vi "探头数据读取.vi"(11 "编号":string) -> ()   [LabVIEW 2022 SP3, in "斯坦道多参数.lvlib"]
panel:
  out "日期/时间字符串 2":string
  out "日期/时间字符串":string
  out "运行状态":u16(ring) items=["空闲", "水样测试", "标样核查"]
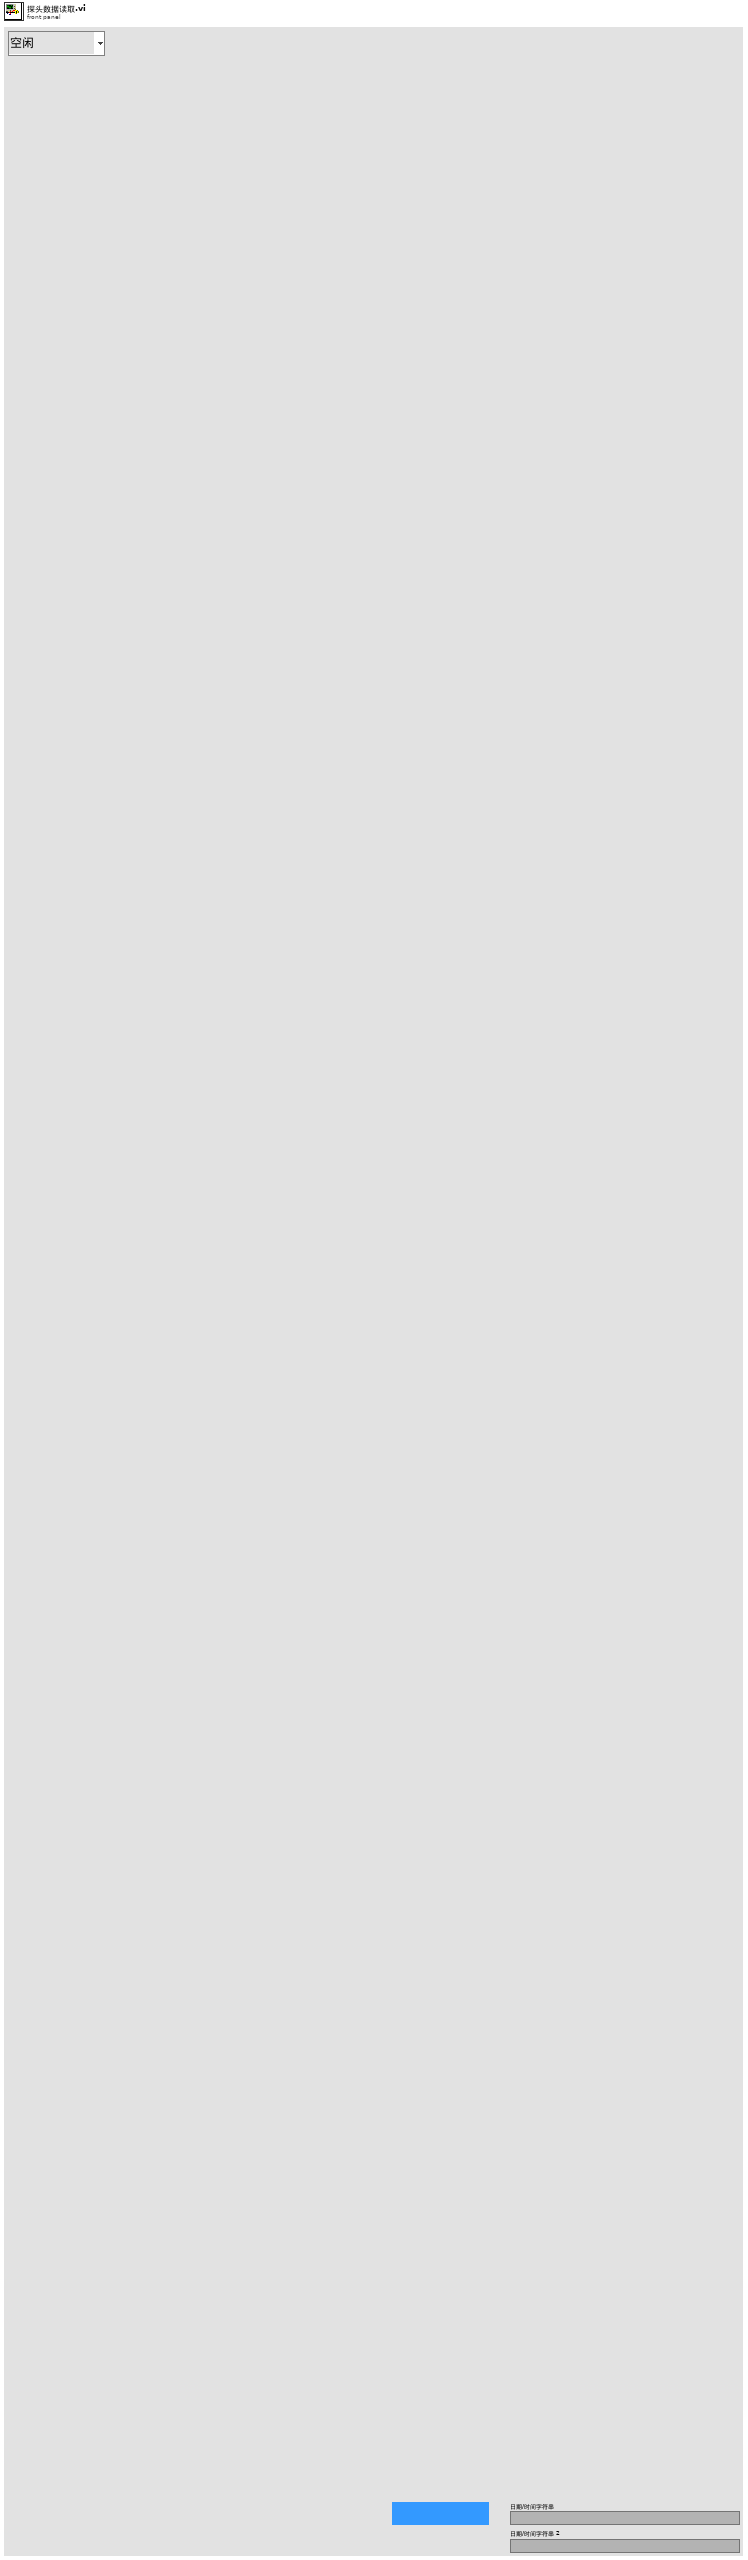
[diagram p1: front panel]
types:
  T1 = typedef "斯坦道多参数.lvlib/通知队列类型.ctl" = enum16{"pH", "DO", "DO2", "Cond", "Turb", "ORP", "叶绿素a", "藻密度", "COD", "氯化物", "氨氮", "水中油", "悬浮物", "余氯"}
  T2 = cluster{"温度测量值":sgl, "测量值":sgl, "温度偏移修正值":sgl, "信号值":sgl, "数据标识":string}
  T3 = cluster{"温度测量值":sgl, "DO%":sgl, "DOmg/L":sgl, "温度偏移修正值":sgl, "数据标识mg/L":string, "数据标识%":string}
  T4 = cluster{"水温 (℃)":cluster{"量程下限":dbl, "量程上限":dbl}, "DO (mg/L)":cluster{"量程下限":dbl, "量程上限":dbl}, "DO (%)":cluster{"量程下限":dbl, "量程上限":dbl}, "pH":cluster{"量程下限":dbl, "量程上限":dbl}, "电导率 (μS/cm)":cluster{"量程下限":dbl, "量程上限":dbl}, "盐度":cluster{"量程下限":dbl, "量程上限":dbl}, "浊度 (NTU)":cluster{"量程下限":dbl, "量程上限":dbl}, "叶绿素a (μg/L)":cluster{"量程下限":dbl, "量程上限":dbl}, "藻密度 (cells/mL)":cluster{"量程下限":dbl, "量程上限":dbl}, "ORP (mV)":cluster{"量程下限":dbl, "量程上限":dbl}, "氯化物（mg/L）":cluster{"量程下限":dbl, "量程上限":dbl}, "COD":cluster{"量程下限":dbl, "量程上限":dbl}, "氨氮":cluster{"量程下限":dbl, "量程上限":dbl}, "水中油":cluster{"量程下限":dbl, "量程上限":dbl}, "悬浮物":cluster{"量程下限":dbl, "量程上限":dbl}, "余氯":cluster{"量程下限":dbl, "量程上限":dbl}}
  T5 = cluster{"CH":u16, "监测值":dbl, "信号值":sgl, "数据标识":string}
  T6 = typedef "斯坦道多参数.lvlib/探头类型.ctl" = enum16{"禹山", "国弘", "纳清", "STD"}
  T7 = cluster{"pH探头选择":T6, "DO探头选择":T6, "电导率探头选择":T6, "浊度探头选择":T6, "悬浮物探头选择":T6, "叶绿素a探头选择":T6, "蓝绿藻探头选择":T6, "orp探头选择":T6, "COD探头选择":T6, "DO2探头选择":T6, "氨氮探头选择":T6, "水中油探头选择":T6, "余氯探头选择":T6}
  T8 = cluster{"电极状态标志":u16, "电极型号标志":u16, "酸碱度测量值":sgl, "温度测量值":sgl, "酸碱度信号值":sgl, "温度信号值":sgl, "酸碱度偏移修正值":sgl, "温度偏移修正值":sgl, "手动温度补偿值":sgl, "酸碱度电极零点":sgl, "酸碱度电极斜率":sgl, "第1点标准值记录":sgl, "第1点信号值记录":sgl, "第1点温度值记录":sgl, "第2点标准值记录":sgl, "第2点信号值记录":sgl, "第2点温度值记录":sgl, "命令滤波设定":u16, "温度模式":enum16{"ATC", "MTC"}, "生产批次":u16, "电极序号":u16, "串口地址":u16, "串口波特率":enum16{"9600", "19200", "115200"}, "串口校验位":enum16{"NONE", "ODD", "EVEN"}, "串口停止位":enum16{"1bit", "2bit"}, "第一点标准值":sgl, "第二点标准值":sgl}
  T9 = cluster{"报警码":u16, "pH数值":sgl, "0X0003_NC":sgl, "温度数据":sgl, "pH原始信号 mv":sgl, "0X0009_NC":string, "产品名称":string, "序列号":string, "硬件版本":string, "软件版本":string, "通讯地址":u16, "波特率":u16, "设备类型":u16, "0X0026_NC":string, "第一点原始数据":sgl, "第一点校准数据":sgl, "第二点原始数据":sgl, "第二点校准数据":sgl, "探头校准命令":u16, "温度校准参数":sgl, "温度校准命令":u16}
  T10 = cluster{"电极状态标志":u16, "电极型号标志":u16, "电导率测量值":sgl, "温度测量值":sgl, "电导率信号值":sgl, "温度信号值":sgl, "温度补偿系数":sgl, "电导率偏移修正值":sgl, "温度偏移修正值":sgl, "手动温度补偿值":sgl, "电导率电极零点":sgl, "电导率电极斜率":sgl, "命令滤波设定":u16, "温度模式":enum16{"ATC", "MTC"}, "生产批次":u16, "电极序号":u16, "串口地址":u16, "串口波特率":enum16{"9600", "19200", "115200"}, "串口校验位":enum16{"NONE", "ODD", "EVEN"}, "串口停止位":enum16{"1bit", "2bit"}, "第一点标准值":sgl, "第二点标准值":sgl}
  T11 = cluster{"报警码":u16, "电导率数据（uS/cm）":sgl, "0x0003 NC":sgl, "温度数据":sgl, "电导率原始信号电阻":sgl, "当前量程":u16, "温度补偿系数":sgl, "0X0009_NC":string, "产品名称":string, "序列号":string, "硬件版本":string, "软件版本":string, "通讯地址":u16, "波特率":u16, "设备类型":u16, "0X0026_NC":string, "第一点原始数据":sgl, "第一点校准数据":sgl, "0X0035_NC":sgl, "0X0037_NC":sgl, "探头校准命令":u16, "温度校准参数":sgl, "温度校准命令":u16}
  T12 = cluster{"电极状态标志":u16, "电极型号标志":u16, "溶解氧测量值":sgl, "温度测量值":sgl, "溶解氧饱和度值":sgl, "盐度补偿值":sgl, "大气压补偿值":sgl, "溶解氧偏移修正值":sgl, "温度偏移修正值":sgl, "手动温度补偿值":sgl, "溶解氧电极零点":sgl, "溶解氧电极斜率":sgl, "第1点标准值记录":sgl, "第1点信号值记录":sgl, "第1点温度值记录":sgl, "第2点标准值记录":sgl, "第2点信号值记录":sgl, "第2点温度值记录":sgl, "命令滤波设定":u16, "温度模式":enum16{"ATC", "MTC"}, "生产批次":u16, "电极序号":u16, "串口地址":u16, "串口波特率":enum16{"9600", "19200", "115200"}, "串口校验位":enum16{"NONE", "ODD", "EVEN"}, "串口停止位":enum16{"1bit", "2bit"}, "第一点标准值":sgl, "第二点标准值":sgl}
  T13 = cluster{"报警码":u16, "溶解氧数值（mg/L）":sgl, "溶解氧数据（%）":sgl, "温度数据":sgl, "溶解氧原始信号 nA":sgl, "大气压力":sgl, "盐度":sgl, "0X0009_NC":string, "产品名称":string, "序列号":string, "硬件版本":string, "软件版本":string, "通讯地址":u16, "波特率":u16, "设备类型":u16, "0X0026_NC":string, "第一点原始数据":sgl, "0X0033 NC":sgl, "第二点原始数据":sgl, "0X0037 NC":sgl, "探头校准命令":u16, "温度校准参数":sgl, "温度校准命令":u16}
  T14 = cluster{"电极状态标志":u16, "电极型号标志":u16, "浊度测量值":sgl, "温度测量值":sgl, "浊度信号值":sgl, "浊度偏移修正值":sgl, "温度偏移修正值":sgl, "手动温度补偿值":sgl, "浊度电极零点":sgl, "浊度电极斜率":sgl, "清洁周期":u16, "命令滤波设定":u16, "温度模式":enum16{"ATC", "MTC"}, "生产批次":u16, "电极序号":u16, "串口地址":u16, "串口波特率":enum16{"9600", "19200", "115200"}, "串口校验位":enum16{"NONE", "ODD", "EVEN"}, "串口停止位":enum16{"1bit", "2bit"}, "第一点标准值":sgl, "第二点标准值":sgl, "第三点标准值":sgl}
  T15 = cluster{"报警码":u16, "浊度数值 NTU":sgl, "温度数据":sgl, "原始光强数值":u16, "量程":u16, "平均次数":u16, "清扫模式":u16, "清扫次数":u16, "清扫间隔分钟":u16, "0X000B_NC":string, "产品名称":string, "序列号":string, "硬件版本":string, "软件版本":string, "通讯地址":u16, "波特率":u16, "设备类型":u16, "0X0026_NC":string, "校准量程":u16, "第一点原始光强":u16, "第一点校准数据":sgl, "第二点原始光强":u16, "第二点校准数据":sgl, "第三点原始光强":u16, "第三点校准数据":sgl, "探头校准命令":u16, "温度校准参数":sgl, "温度校准命令":u16}
  T16 = cluster{"电极状态标志":u16, "电极型号标志":u16, "测量值":sgl, "温度测量值":sgl, "信号值":sgl, "温度信号值":sgl, "000AH_NC":sgl, "偏移修正值":sgl, "温度偏移修正值":sgl, "手动温度补偿值":sgl, "命令滤波设定":u16, "温度模式":enum16{"ATC", "MTC"}, "生产批次":u16, "传感器序号":u16, "串口地址":u16, "串口波特率":enum16{"9600", "19200", "115200"}, "串口校验位":enum16{"NONE", "ODD", "EVEN"}, "串口停止位":enum16{"1bit", "2bit"}}
  T17 = cluster{"报警码":u16, "叶绿素a":sgl, "温度数据":sgl, "原始光强数值":u16, "量程":u16, "平均次数":u16, "清扫模式":u16, "清扫次数":u16, "清扫间隔分钟":u16, "0X000B_NC":string, "产品名称":string, "序列号":string, "硬件版本":string, "软件版本":string, "通讯地址":u16, "波特率":u16, "设备类型":u16, "0X0026_NC":string, "校准量程":u16, "第一点原始光强":u16, "第一点校准数据":sgl, "第二点原始光强":u16, "第二点校准数据":sgl, "第三点原始光强":u16, "第三点校准数据":sgl, "探头校准命令":u16, "温度校准参数":sgl, "温度校准命令":u16}
  T18 = cluster{"报警码":u16, "蓝绿藻":sgl, "温度数据":sgl, "原始光强数值":u16, "0X0006_NC":u16, "平均次数":u16, "清扫模式":u16, "清扫次数":u16, "清扫间隔分钟":u16, "0X000B_NC":string, "产品名称":string, "序列号":string, "硬件版本":string, "软件版本":string, "通讯地址":u16, "波特率":u16, "设备类型":u16, "0X0026_NC":string, "0X0030_NC":u16, "第一点原始光强":u16, "第一点校准数据":sgl, "第二点原始光强":u16, "第二点校准数据":sgl, "第三点原始光强":u16, "第三点校准数据":sgl, "探头校准命令":u16, "温度校准参数":sgl, "温度校准命令":u16}
  T19 = cluster{"电极状态标志":u16, "电极型号标志":u16, "COD测量值":sgl, "浊度测量值":sgl, "COD信号值":sgl, "浊度信号值":sgl, "温度测量值":sgl, "COD偏移修正值":sgl, "浊度偏移修正值":sgl, "COD水样校正值":sgl, "温度偏移修正值":sgl, "COD零点系数":sgl, "COD斜率系数":sgl, "浊度零点系数":sgl, "浊度斜率系数":sgl, "COD测值K值":sgl, "浊度测值K值":sgl, "浊度补偿COD系数值":sgl, "COD温度补偿系数值 ":sgl, "测量周期":u16, "清洗周期":u16, "命令寄存器":u16, "数字滤波设定":u16, "温度模式":enum16{"AUTO", "OFF"}, "生产批次":u16, "电极序号":u16, "串口地址":u16, "串口波特率":enum16{"9600", "19200", "115200"}, "串口校验位":enum16{"NONE", "ODD", "EVEN"}, "串口停止位":enum16{"1bit", "2bit"}, "第一点校正指令":u16, "第一点标准值":sgl, "第二点校正指令":u16, "第二点标准值":sgl, "第三点校正指令":u16, "第三点标准值":sgl, "COD吸光度":sgl, "浊度吸光度":sgl, "温度信号值":sgl}
  T20 = cluster{"电极状态标志":u16, "电极型号标志":u16, "测量值":sgl, "温度测量值":sgl, "信号值":sgl, "温度信号值":sgl, "偏移修正值":sgl, "温度偏移修正值":sgl, "手动温度补偿值":sgl, "电极零点":sgl, "电极斜率":sgl, "第1点标准值记录":sgl, "第1点信号值记录":sgl, "第1点温度值记录":sgl, "第2点标准值记录":sgl, "第2点信号值记录":sgl, "第2点温度值记录":sgl, "命令滤波设定":u16, "温度模式":enum16{"ATC", "MTC"}, "生产批次":u16, "电极序号":u16, "串口地址":u16, "串口波特率":enum16{"9600", "19200", "115200"}, "串口校验位":enum16{"NONE", "ODD", "EVEN"}, "串口停止位":enum16{"1bit", "2bit"}, "第一点标准值":sgl, "第二点标准值":sgl}
  T21 = cluster{"电极状态标志":u16, "电极型号标志":u16, "测量值":sgl, "温度测量值":sgl, "信号值":sgl, "水中油B值":sgl, "温度B值":sgl, "水中油零点系数":sgl, "水中油斜率系数":sgl, "水中油K值":sgl, "空白电位值":sgl, "温度信号值":sgl, "温度补偿系数":sgl, "测量档位":u16, "清洁周期":u16, "命令寄存器":u16, "数位滤波设定":u16, "温度模式":enum16{"ATC", "MTC"}, "生产批次":u16, "电极序号":u16, "串口地址":u16, "串口波特率":enum16{"9600", "19200", "115200"}, "串口校验位":enum16{"NONE", "ODD", "EVEN"}, "串口停止位":enum16{"1bit", "2bit"}, "第一点校正指令":u16, "第一点标准值":sgl, "第二点校正指令":u16, "第二点标准值":sgl, "第三点校正指令":u16, "第三点标准值":sgl}
  T22 = cluster{"余氯值":sgl, "温度值":sgl, "温度电压_mv":sgl, "氯电压_mv":dbl, "pH补偿值":dbl, "氯偏置":dbl, "温度偏置":dbl, "序列号":string}
  T23 = cluster{"报警码":u16, "参数1数据":sgl, "参数2数据":sgl, "参数3数据":sgl, "参数4数据":sgl, "温度数据":sgl, "参数1原始信号":sgl, "参数2原始信号":sgl, "参数3原始信号":sgl, "参数4原始信号":sgl, "序列号":string, "硬件版本":string, "软件版本":string, "通讯地址":u16, "波特率":u16, "设备类型":u16, "0X0026_NC":string, "校准参数类型":u16, "第一点原始数据":sgl, "第一点校准数据":sgl, "第二点原始数据":sgl, "第二点校准数据":sgl, "探头校准命令":u16, "温度校准参数":sgl, "温度校准命令":u16}
  T24 = cluster{"ph":bool, "DO":bool, "Cond":bool, "Turb":bool, "叶绿素a":bool, "藻密度":bool, "ORP":bool, "cod":bool, "DO2":bool, "氯化物":bool, "氨氮":bool, "水中油":bool, "悬浮物":bool, "余氯":bool}
  T25 = cluster{"ph":bool, "DO":bool, "Cond":bool, "Turb":bool, "叶绿素a":bool, "藻密度":bool, "ORP":bool, "COD":bool, "DO2":bool, "氯化物":bool, "氨氮":bool, "水中油":bool, "悬浮物":bool, "余氯":bool}
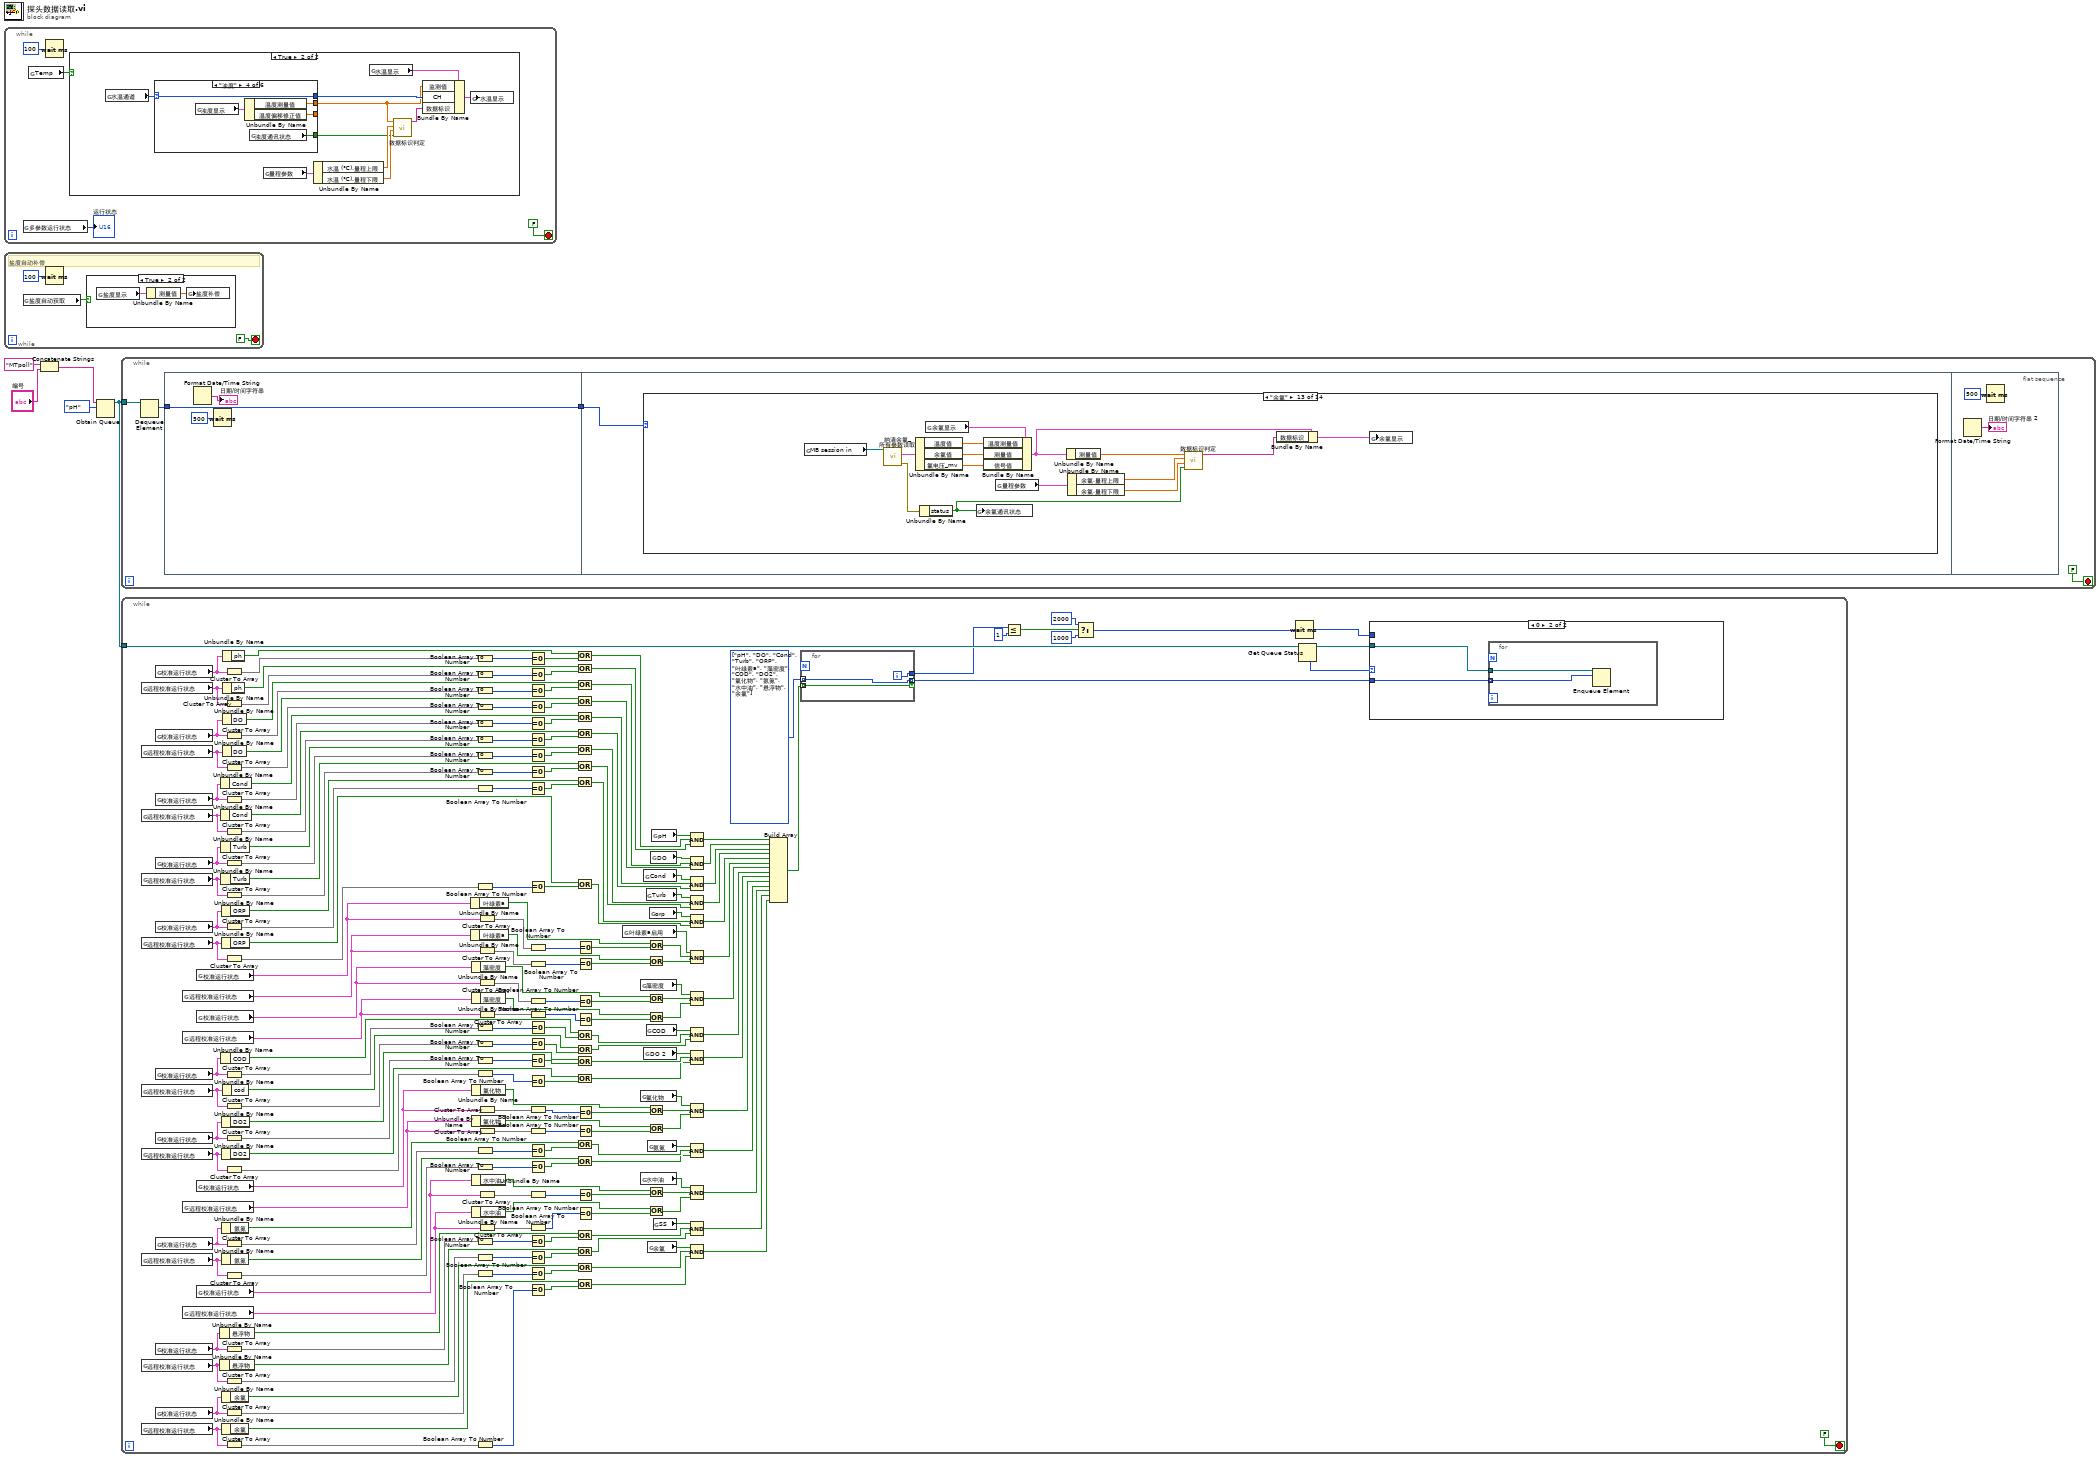
[diagram p0: block diagram]
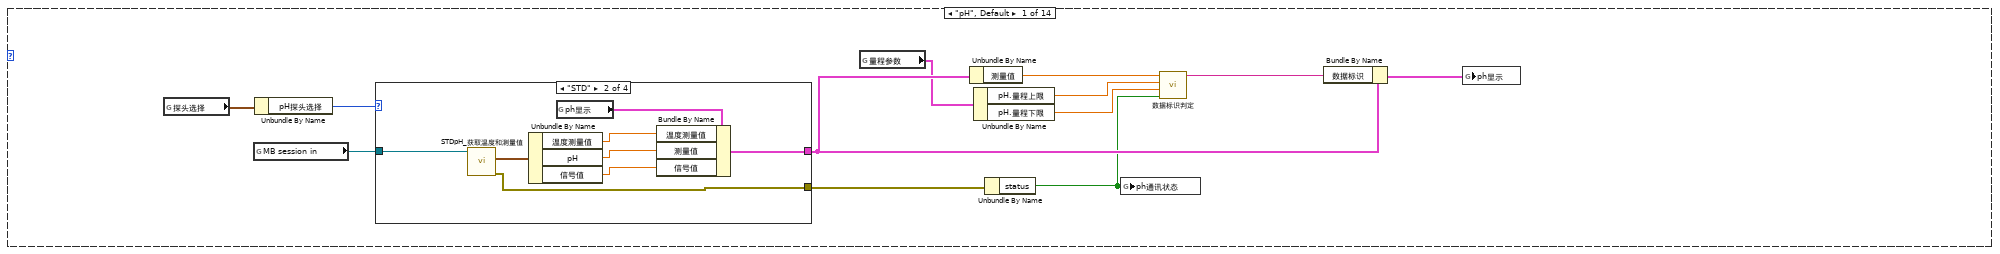
[diagram p3: hidden frame]
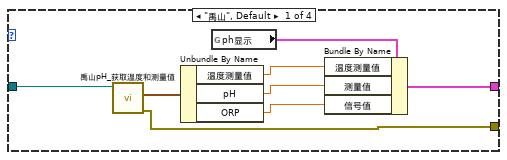
[diagram p4: hidden frame]
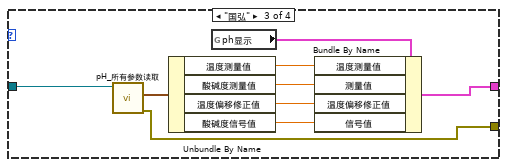
[diagram p5: hidden frame]
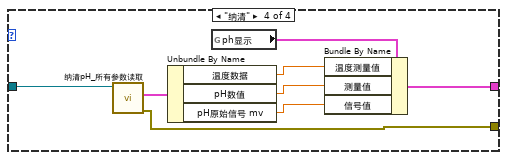
[diagram p6: hidden frame]
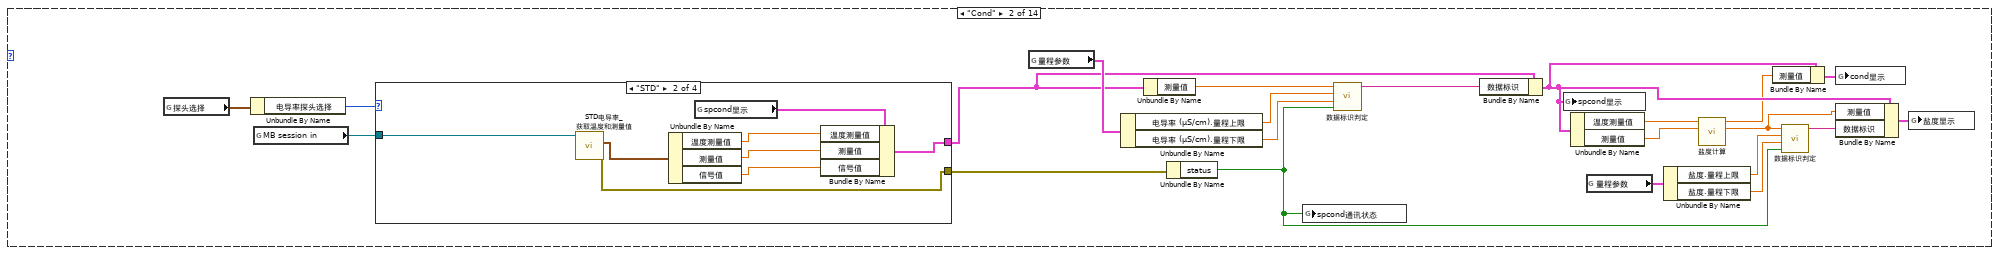
[diagram p7: hidden frame]
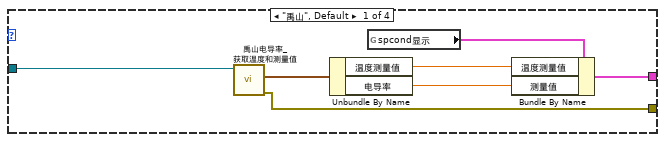
[diagram p8: hidden frame]
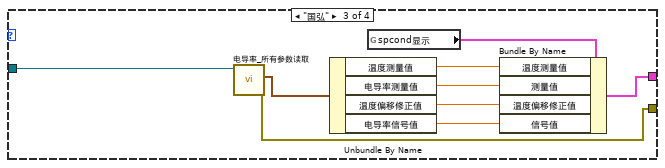
[diagram p9: hidden frame]
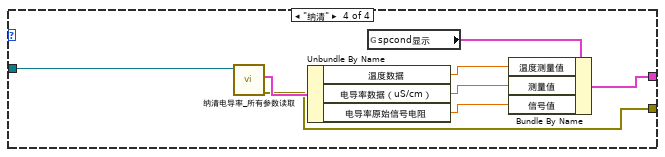
[diagram p10: hidden frame]
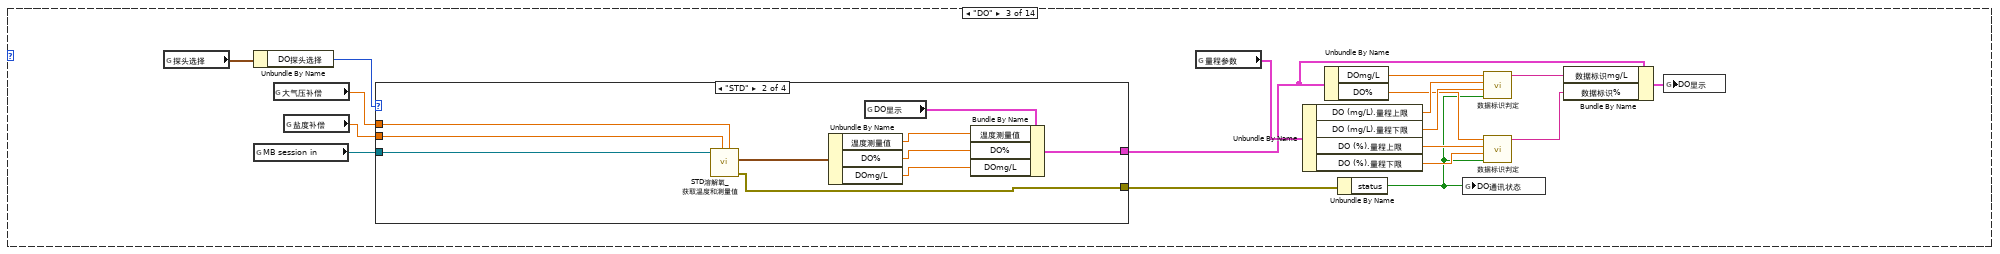
[diagram p11: hidden frame]
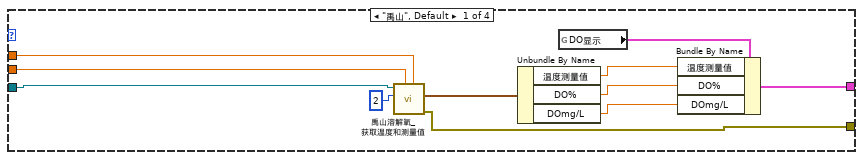
[diagram p12: hidden frame]
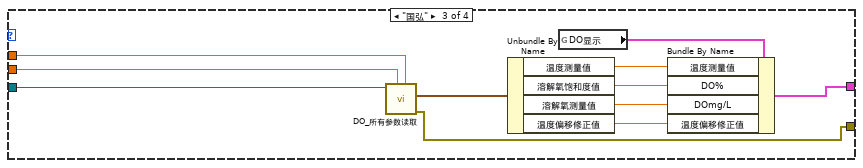
[diagram p13: hidden frame]
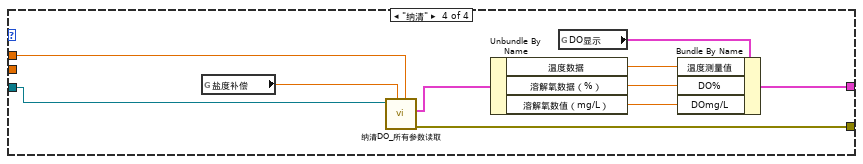
[diagram p14: hidden frame]
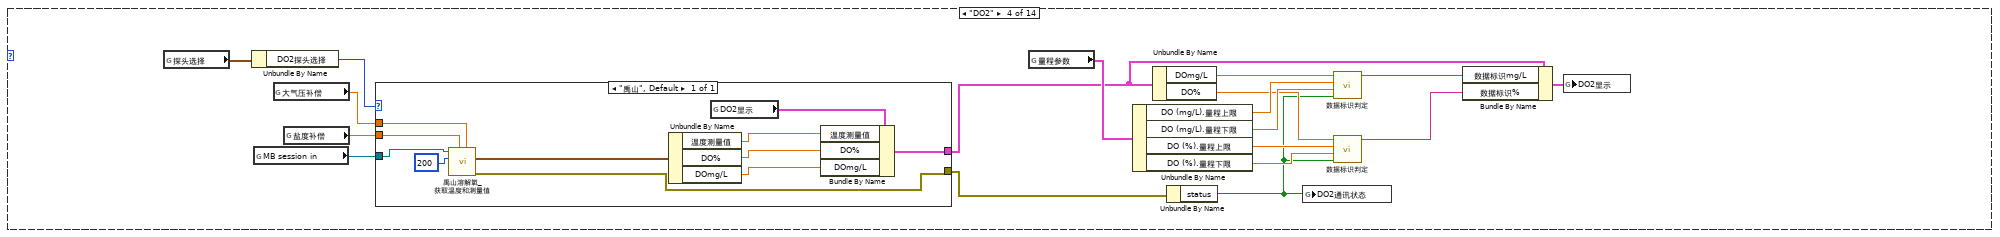
[diagram p15: hidden frame]
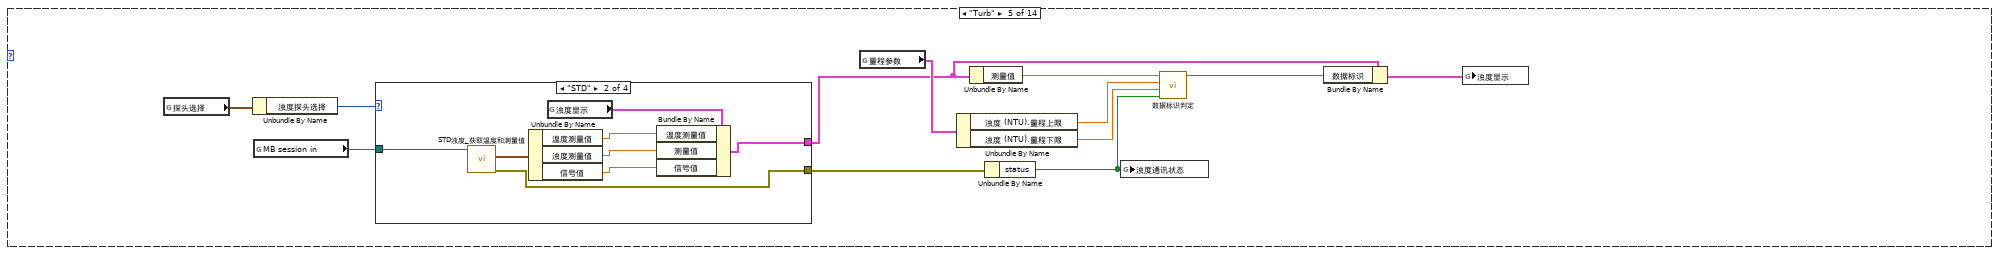
[diagram p16: hidden frame]
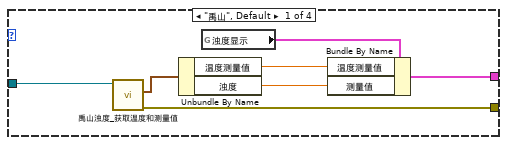
[diagram p17: hidden frame]
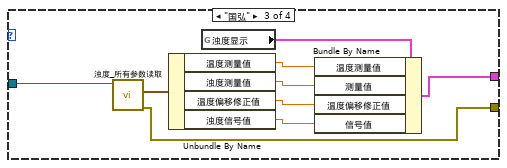
[diagram p18: hidden frame]
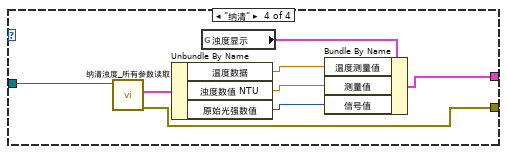
[diagram p19: hidden frame]
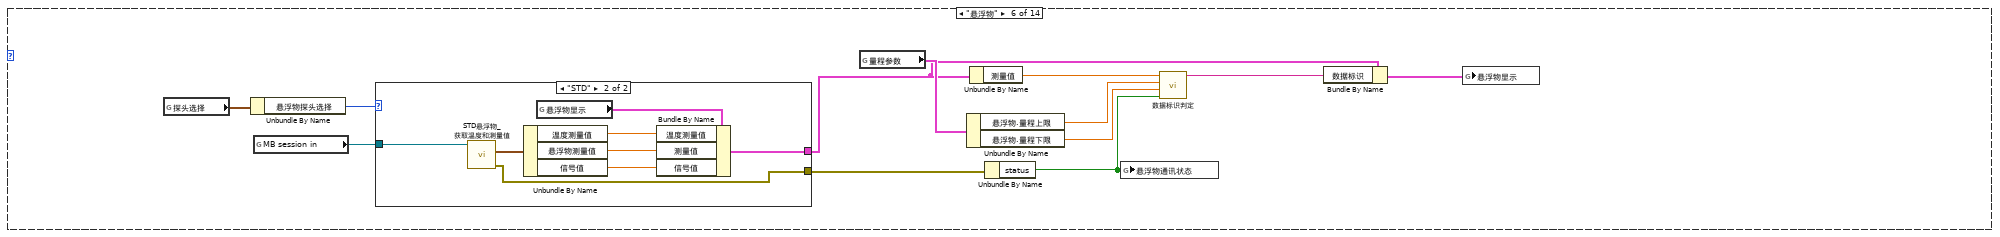
[diagram p20: hidden frame]
diagram:
  n1 = while {
    stop <- FALSE stop-if-true
    n2 = global read "多参数全局变量.vi" "多参数运行状态"() -> (→"运行状态":u16)
    n3 = global read "断电保存变量.vi" "Temp"() -> (w7:bool)
    n4 = Wait (ms)(milliseconds to wait=u32 100 ("等待时间（毫秒）")) -> ()  [unwired: 1 out]
    n5 = case shown="True" w7 {
      frame False {
      }
      frame True {
        n6 = global read "断电保存变量.vi" "水温通道"() -> (w19:enum16{"pH", "DO", "浊度", "电导率", "叶绿素a", "藻密度"})
        n7 = case shown="\"浊度\"" w19 {
          selector: w19 -> [w24 w29 w34 w39 w44 w49]
          tunnel: [w24 w29 w34 w39 w44 w49] -> w18
          tunnel: [w22 w26 w31 w36 w41 w46] -> _
          tunnel: [w23 w27 w32 w37 w42 w47] -> w12
          tunnel: [w20 w25 w30 w35 w40 w45] -> w10
          frame "pH", Default {
            n8 = global read "多参数全局变量.vi" "ph显示"() -> (w21:T2)
            n9 = Unbundle By Name(w21) -> ("温度测量值"=w23:sgl, "温度偏移修正值"=w22:sgl)
            n10 = global read "多参数全局变量.vi" "ph通讯状态"() -> (w20:bool)
          }
          frame "电导率" {
            n11 = global read "多参数全局变量.vi" "spcond显示"() -> (w28:T2)
            n12 = global read "多参数全局变量.vi" "spcond通讯状态"() -> (w25:bool)
            n13 = Unbundle By Name(w28) -> ("温度测量值"=w27:sgl, "温度偏移修正值"=w26:sgl)
          }
          frame "DO" {
            n14 = global read "多参数全局变量.vi" "DO显示"() -> (w33:T3)
            n15 = Unbundle By Name(w33) -> ("温度测量值"=w32:sgl, "温度偏移修正值"=w31:sgl)
            n16 = global read "多参数全局变量.vi" "DO通讯状态"() -> (w30:bool)
          }
          frame "浊度" {
            n17 = global read "多参数全局变量.vi" "浊度显示"() -> (w38:T2)
            n18 = Unbundle By Name(w38) -> ("温度测量值"=w37:sgl, "温度偏移修正值"=w36:sgl)
            n19 = global read "多参数全局变量.vi" "浊度通讯状态"() -> (w35:bool)
          }
          frame "叶绿素a" {
            n20 = global read "多参数全局变量.vi" "叶绿素a显示"() -> (w43:T2)
            n21 = global read "多参数全局变量.vi" "叶绿素a通讯状态"() -> (w40:bool)
            n22 = Unbundle By Name(w43) -> ("温度测量值"=w42:sgl, "温度偏移修正值"=w41:sgl)
          }
          frame "藻密度" {
            n23 = global read "多参数全局变量.vi" "藻密度显示"() -> (w48:T2)
            n24 = global read "多参数全局变量.vi" "藻密度通讯状态"() -> (w45:bool)
            n25 = Unbundle By Name(w48) -> ("温度测量值"=w47:sgl, "温度偏移修正值"=w46:sgl)
          }
        }
        n26 = global read "断电保存变量.vi" "量程参数"() -> (w15:T4)
        n27 = Unbundle By Name(w15) -> ("水温 (℃).量程上限"=w13:dbl, "水温 (℃).量程下限"=w14:dbl)
        n28 = global read "多参数全局变量.vi" "水温显示"() -> (w16:T5)
        n29 = call "数据标识判定.vi"("通讯故障"=w10, "量程下限"=w14, "量程上限"=w13, "测量值"=w12) -> ("数据标识"=w11:string)  [unwired: 7 in]
        n30 = Bundle By Name(cluster=w16, "监测值"=w12, "CH"=w18, "数据标识"=w11) -> (w17:T5)
        n31 = global write "多参数全局变量.vi" "水温显示"(w17) -> ()
      }
    }
  }
  n32 = while {
    stop <- FALSE stop-if-true
    # "盐度自动补偿"
    n33 = global read "断电保存变量.vi" "盐度自动获取"() -> (w51:bool)
    n34 = Wait (ms)(milliseconds to wait=u32 100 ("等待时间（毫秒）")) -> ()  [unwired: 1 out]
    n35 = case shown="True" w51 {
      frame False {
      }
      frame True {
        n36 = global read "多参数全局变量.vi" "盐度显示"() -> (w54:T2)
        n37 = Unbundle By Name(w54) -> ("测量值"=w53:sgl)
        n38 = global write "断电保存变量.vi" "盐度补偿"(w53) -> ()
      }
    }
  }
  n39 = Concatenate Strings("MTpoll" ("名称（未命名）"), "编号") -> (w3:string)
  n40 = Obtain Queue(name (unnamed)=w3, element data type=通知队列类型."pH" ("枚举")) -> (queue out=w1:refnum<queue>)  [unwired: 3 in, 2 out]
  n41 = while {
    tunnel: w1 -> [w58]
    stop <- FALSE stop-if-true
    n42 = Dequeue Element(queue=w58) -> (element=w57:T1)  [unwired: 2 in, 3 out]
    n43 = flat-sequence {
      tunnel: w57 -> [w61]
      tunnel: [w61] -> w55
      tunnel: w55 -> [w62]
      frame #0 {
        n44 = Format Date/Time String() -> (date/time string=→"日期/时间字符串":string)  [unwired: 3 in]
        n45 = Wait (ms)(milliseconds to wait=u32 500 ("等待时间（毫秒）")) -> ()  [unwired: 1 out]
      }
      frame #1 {
        n46 = case shown="\"余氯\"" w62 {
          frame "pH", Default {
            n47 = global read "断电保存变量.vi" "探头选择"() -> (w74:T7)
            n48 = global read "多参数全局变量.vi" "MB session in"() -> (w72:refnum<class "MB_Master.lvclass">)
            n49 = Unbundle By Name(w74) -> ("pH探头选择"=w73:T6)
            n50 = case shown="\"STD\"" w73 {
              tunnel: w72 -> [w82 w90 w99 w105]
              tunnel: [w81 w89 w98 w103] -> w71
              tunnel: [w79 w87 w95 w106] -> w70
              frame "禹山", Default {
                n51 = call "禹山pH_获取温度和测量值.vi"("MB session in"=w82) -> ("error out"=w81:errorcluster, "输出值"=w78:cluster{"温度测量值":sgl, "ORP":sgl, "pH":sgl})  [unwired: 8 in, 1 out]
                n52 = Unbundle By Name(w78) -> ("温度测量值"=w77:sgl, "pH"=w76:sgl, "ORP"=w75:sgl)
                n53 = global read "多参数全局变量.vi" "ph显示"() -> (w80:T2)
                n54 = Bundle By Name(cluster=w80, "温度测量值"=w77, "测量值"=w76, "信号值"=w75) -> (w79:T2)
              }
              frame "STD" {
                n55 = call "STDpH_获取温度和测量值.vi"("MB session in"=w90) -> ("error out"=w89:errorcluster, "STDpH"=w83:cluster{"温度测量值":sgl, "pH":sgl, "信号值":sgl})  [unwired: 8 in, 1 out]
                n56 = Unbundle By Name(w83) -> ("温度测量值"=w86:sgl, "pH"=w85:sgl, "信号值"=w84:sgl)
                n57 = global read "多参数全局变量.vi" "ph显示"() -> (w88:T2)
                n58 = Bundle By Name(cluster=w88, "温度测量值"=w86, "测量值"=w85, "信号值"=w84) -> (w87:T2)
              }
              frame "国弘" {
                n59 = call "pH_所有参数读取.vi"("MB session in"=w99) -> ("error out"=w98:errorcluster, "输出值"=w97:T8)  [unwired: 8 in, 1 out]
                n60 = Unbundle By Name(w97) -> ("温度测量值"=w92:sgl, "酸碱度测量值"=w93:sgl, "温度偏移修正值"=w94:sgl, "酸碱度信号值"=w91:sgl)
                n61 = global read "多参数全局变量.vi" "ph显示"() -> (w96:T2)
                n62 = Bundle By Name(cluster=w96, "温度测量值"=w92, "测量值"=w93, "温度偏移修正值"=w94, "信号值"=w91) -> (w95:T2)
              }
              frame "纳清" {
                n63 = call "纳清pH_所有参数读取.vi"("MB session in"=w105) -> ("error out"=w103:errorcluster, "输出值"=w104:T9)  [unwired: 8 in, 1 out]
                n64 = Unbundle By Name(w104) -> ("温度数据"=w102:sgl, "pH数值"=w101:sgl, "pH原始信号 mv"=w100:sgl)
                n65 = global read "多参数全局变量.vi" "ph显示"() -> (w107:T2)
                n66 = Bundle By Name(cluster=w107, "温度测量值"=w102, "测量值"=w101, "信号值"=w100) -> (w106:T2)
              }
            }
            n67 = global read "断电保存变量.vi" "量程参数"() -> (w69:T4)
            n68 = Unbundle By Name(w70) -> ("测量值"=w68:sgl)
            n69 = Unbundle By Name(w69) -> ("pH.量程上限"=w67:dbl, "pH.量程下限"=w66:dbl)
            n70 = Unbundle By Name(w71) -> ("status"=w65:bool)
            n71 = global write "多参数全局变量.vi" "ph通讯状态"(w65) -> ()
            n72 = call "数据标识判定.vi"("通讯故障"=w65, "量程下限"=w66, "量程上限"=w67, "测量值"=w68) -> ("数据标识"=w63:string)  [unwired: 7 in]
            n73 = Bundle By Name(cluster=w70, "数据标识"=w63) -> (w64:T2)
            n74 = global write "多参数全局变量.vi" "ph显示"(w64) -> ()
          }
          frame "Cond" {
            n75 = global read "断电保存变量.vi" "探头选择"() -> (w129:T7)
            n76 = Unbundle By Name(w129) -> ("电导率探头选择"=w128:T6)
            n77 = global read "多参数全局变量.vi" "MB session in"() -> (w127:refnum<class "MB_Master.lvclass">)
            n78 = case shown="\"STD\"" w128 {
              tunnel: w127 -> [w136 w144 w153 w157]
              tunnel: [w130 w138 w151 w160] -> w122
              tunnel: [w135 w143 w150 w155] -> w126
              frame "禹山", Default {
                n79 = call "禹山电导率_获取温度和测量值.vi"("MB session in"=w136) -> ("error out"=w135:errorcluster, "输出值"=w133:cluster{"温度测量值":sgl, "电导率":sgl, "错误标志":u16})  [unwired: 8 in, 1 out]
                n80 = Unbundle By Name(w133) -> ("温度测量值"=w132:sgl, "电导率"=w131:sgl)
                n81 = global read "多参数全局变量.vi" "spcond显示"() -> (w134:T2)
                n82 = Bundle By Name(cluster=w134, "温度测量值"=w132, "测量值"=w131) -> (w130:T2)
              }
              frame "STD" {
                n83 = call "STD电导率_获取温度和测量值.vi"("MB session in"=w144) -> ("error out"=w143:errorcluster, "STDspcond"=w141:cluster{"温度测量值":sgl, "测量值":sgl, "信号值":sgl})  [unwired: 8 in, 1 out]
                n84 = Unbundle By Name(w141) -> ("温度测量值"=w140:sgl, "测量值"=w139:sgl, "信号值"=w137:sgl)
                n85 = global read "多参数全局变量.vi" "spcond显示"() -> (w142:T2)
                n86 = Bundle By Name(cluster=w142, "温度测量值"=w140, "测量值"=w139, "信号值"=w137) -> (w138:T2)
              }
              frame "国弘" {
                n87 = call "电导率_所有参数读取.vi"("MB session in"=w153) -> ("error out"=w150:errorcluster, "输出值"=w149:T10)  [unwired: 8 in, 1 out]
                n88 = Unbundle By Name(w149) -> ("温度测量值"=w148:sgl, "电导率测量值"=w147:sgl, "温度偏移修正值"=w146:sgl, "电导率信号值"=w145:sgl)
                n89 = global read "多参数全局变量.vi" "spcond显示"() -> (w152:T2)
                n90 = Bundle By Name(cluster=w152, "温度测量值"=w148, "测量值"=w147, "温度偏移修正值"=w146, "信号值"=w145) -> (w151:T2)
              }
              frame "纳清" {
                n91 = call "纳清电导率_所有参数读取.vi"("MB session in"=w157) -> ("error out"=w155:errorcluster, "输出值"=w156:T11)  [unwired: 8 in, 1 out]
                n92 = Unbundle By Name(w156) -> ("温度数据"=w159:sgl, "电导率数据（uS/cm）"=w158:sgl, "电导率原始信号电阻"=w154:sgl)
                n93 = global read "多参数全局变量.vi" "spcond显示"() -> (w161:T2)
                n94 = Bundle By Name(cluster=w161, "温度测量值"=w159, "测量值"=w158, "信号值"=w154) -> (w160:T2)
              }
            }
            n95 = global read "断电保存变量.vi" "量程参数"() -> (w125:T4)
            n96 = Unbundle By Name(w125) -> ("电导率 (μS/cm).量程上限"=w124:dbl, "电导率 (μS/cm).量程下限"=w123:dbl)
            n97 = Unbundle By Name(w122) -> ("测量值"=w121:sgl)
            n98 = Unbundle By Name(w126) -> ("status"=w118:bool)
            n99 = global write "多参数全局变量.vi" "spcond通讯状态"(w118) -> ()
            n100 = call "数据标识判定.vi"("通讯故障"=w118, "量程下限"=w123, "量程上限"=w124, "测量值"=w121) -> ("数据标识"=w119:string)  [unwired: 7 in]
            n101 = Bundle By Name(cluster=w122, "数据标识"=w119) -> (w120:T2)
            n102 = global write "多参数全局变量.vi" "spcond显示"(w120) -> ()
            n103 = Unbundle By Name(w120) -> ("温度测量值"=w117:sgl, "测量值"=w116:sgl)
            n104 = global read "断电保存变量.vi" "量程参数"() -> (w110:T4)
            n105 = Unbundle By Name(w110) -> ("盐度.量程上限"=w111:dbl, "盐度.量程下限"=w112:dbl)
            n106 = call "盐度计算.vi"("spCond"=w116, "Temp"=w117) -> ("saltresult"=w109:dbl, "cond"=w115:dbl)  [unwired: 8 in]
            n107 = Bundle By Name(cluster=w120, "测量值"=w115) -> (w114:T2)
            n108 = call "数据标识判定.vi"("通讯故障"=w118, "量程下限"=w112, "量程上限"=w111, "测量值"=w109) -> ("数据标识"=w108:string)  [unwired: 7 in]
            n109 = global write "多参数全局变量.vi" "cond显示"(w114) -> ()
            n110 = Bundle By Name(cluster=w120, "测量值"=w109, "数据标识"=w108) -> (w113:T2)
            n111 = global write "多参数全局变量.vi" "盐度显示"(w113) -> ()
          }
          frame "DO" {
            n112 = global read "断电保存变量.vi" "探头选择"() -> (w179:T7)
            n113 = Unbundle By Name(w179) -> ("DO探头选择"=w178:T6)
            n114 = global read "多参数全局变量.vi" "MB session in"() -> (w177:refnum<class "MB_Master.lvclass">)
            n115 = global read "断电保存变量.vi" "大气压补偿"() -> (w162:dbl)
            n116 = global read "断电保存变量.vi" "盐度补偿"() -> (w163:dbl)
            n117 = case shown="\"STD\"" w178 {
              tunnel: w177 -> [w190 w200 w211 w216]
              tunnel: [w188 w198 w209 w220] -> w170
              tunnel: [w180 w191 w204 w214] -> w176
              tunnel: w163 -> [w182 w193 w202 _]
              tunnel: w162 -> [w181 w192 w201 w212]
              frame "禹山", Default {
                n118 = call "禹山溶解氧_获取温度和测量值.vi"("大气压补偿"=w181, "盐度补偿"=w182, "salve ID"=u16 2, "MB session in"=w190) -> ("error out"=w180:errorcluster, "输出值"=w184:cluster{"温度测量值":sgl, "DO%":sgl, "DOmg/L":sgl})  [unwired: 5 in, 1 out]
                n119 = Unbundle By Name(w184) -> ("温度测量值"=w187:sgl, "DO%"=w186:sgl, "DOmg/L"=w185:sgl)
                n120 = global read "多参数全局变量.vi" "DO显示"() -> (w189:T3)
                n121 = Bundle By Name(cluster=w189, "温度测量值"=w187, "DO%"=w186, "DOmg/L"=w185) -> (w188:T3)
              }
              frame "STD" {
                n122 = call "STD溶解氧_获取温度和测量值.vi"("大气压补偿"=w192, "盐度补偿"=w193, "MB session in"=w200) -> ("error out"=w191:errorcluster, "输出值"=w194:cluster{"温度测量值":sgl, "DO%":sgl, "DOmg/L":sgl})  [unwired: 6 in, 1 out]
                n123 = Unbundle By Name(w194) -> ("温度测量值"=w197:sgl, "DO%"=w196:sgl, "DOmg/L"=w195:sgl)
                n124 = global read "多参数全局变量.vi" "DO显示"() -> (w199:T3)
                n125 = Bundle By Name(cluster=w199, "温度测量值"=w197, "DO%"=w196, "DOmg/L"=w195) -> (w198:T3)
              }
              frame "国弘" {
                n126 = call "DO_所有参数读取.vi"("大气压补偿"=w201, "盐度补偿"=w202, "MB session in"=w211) -> ("error out"=w204:errorcluster, "输出值"=w208:T12)  [unwired: 6 in, 1 out]
                n127 = Unbundle By Name(w208) -> ("温度测量值"=w205:sgl, "溶解氧饱和度值"=w206:sgl, "溶解氧测量值"=w207:sgl, "温度偏移修正值"=w203:sgl)
                n128 = global read "多参数全局变量.vi" "DO显示"() -> (w210:T3)
                n129 = Bundle By Name(cluster=w210, "温度测量值"=w205, "DO%"=w206, "DOmg/L"=w207, "温度偏移修正值"=w203) -> (w209:T3)
              }
              frame "纳清" {
                n130 = global read "断电保存变量.vi" "盐度补偿"() -> (w213:dbl)
                n131 = call "纳清DO_所有参数读取.vi"("大气压补偿"=w212, "盐度补偿"=w213, "MB session in"=w216) -> ("error out"=w214:errorcluster, "输出值"=w215:T13)  [unwired: 6 in, 1 out]
                n132 = Unbundle By Name(w215) -> ("温度数据"=w217:sgl, "溶解氧数据（%）"=w218:sgl, "溶解氧数值（mg/L）"=w219:sgl)
                n133 = global read "多参数全局变量.vi" "DO显示"() -> (w221:T3)
                n134 = Bundle By Name(cluster=w221, "温度测量值"=w217, "DO%"=w218, "DOmg/L"=w219) -> (w220:T3)
              }
            }
            n135 = global read "断电保存变量.vi" "量程参数"() -> (w175:T4)
            n136 = Unbundle By Name(w175) -> ("DO (mg/L).量程上限"=w174:dbl, "DO (mg/L).量程下限"=w173:dbl, "DO (%).量程上限"=w172:dbl, "DO (%).量程下限"=w171:dbl)
            n137 = Unbundle By Name(w170) -> ("DOmg/L"=w169:sgl, "DO%"=w168:sgl)
            n138 = Unbundle By Name(w176) -> ("status"=w164:bool)
            n139 = global write "多参数全局变量.vi" "DO通讯状态"(w164) -> ()
            n140 = call "数据标识判定.vi"("通讯故障"=w164, "量程下限"=w173, "量程上限"=w174, "测量值"=w169) -> ("数据标识"=w166:string)  [unwired: 7 in]
            n141 = call "数据标识判定.vi"("通讯故障"=w164, "量程下限"=w171, "量程上限"=w172, "测量值"=w168) -> ("数据标识"=w165:string)  [unwired: 7 in]
            n142 = Bundle By Name(cluster=w170, "数据标识mg/L"=w166, "数据标识%"=w165) -> (w167:T3)
            n143 = global write "多参数全局变量.vi" "DO显示"(w167) -> ()
          }
          frame "DO2" {
            n144 = global read "断电保存变量.vi" "探头选择"() -> (w239:T7)
            n145 = Unbundle By Name(w239) -> ("DO2探头选择"=w238:T6)
            n146 = global read "多参数全局变量.vi" "MB session in"() -> (w237:refnum<class "MB_Master.lvclass">)
            n147 = global read "断电保存变量.vi" "大气压补偿"() -> (w222:dbl)
            n148 = global read "断电保存变量.vi" "盐度补偿"() -> (w223:dbl)
            n149 = case shown="\"禹山\", Default" w238 {
              tunnel: w237 -> [w250]
              tunnel: [w248] -> w230
              tunnel: [w244] -> w236
              tunnel: w223 -> [w241]
              tunnel: w222 -> [w240]
              frame "禹山", Default {
                n150 = call "禹山溶解氧_获取温度和测量值.vi"("大气压补偿"=w240, "盐度补偿"=w241, "salve ID"=u16 200, "MB session in"=w250) -> ("error out"=w244:errorcluster, "输出值"=w243:cluster{"温度测量值":sgl, "DO%":sgl, "DOmg/L":sgl})  [unwired: 5 in, 1 out]
                n151 = Unbundle By Name(w243) -> ("温度测量值"=w247:sgl, "DO%"=w246:sgl, "DOmg/L"=w245:sgl)
                n152 = global read "多参数全局变量.vi" "DO2显示"() -> (w249:T3)
                n153 = Bundle By Name(cluster=w249, "温度测量值"=w247, "DO%"=w246, "DOmg/L"=w245) -> (w248:T3)
              }
            }
            n154 = global read "断电保存变量.vi" "量程参数"() -> (w235:T4)
            n155 = Unbundle By Name(w235) -> ("DO (mg/L).量程上限"=w234:dbl, "DO (mg/L).量程下限"=w233:dbl, "DO (%).量程上限"=w232:dbl, "DO (%).量程下限"=w231:dbl)
            n156 = Unbundle By Name(w230) -> ("DOmg/L"=w229:sgl, "DO%"=w228:sgl)
            n157 = Unbundle By Name(w236) -> ("status"=w224:bool)
            n158 = global write "多参数全局变量.vi" "DO2通讯状态"(w224) -> ()
            n159 = call "数据标识判定.vi"("通讯故障"=w224, "量程下限"=w233, "量程上限"=w234, "测量值"=w229) -> ("数据标识"=w226:string)  [unwired: 7 in]
            n160 = call "数据标识判定.vi"("通讯故障"=w224, "量程下限"=w231, "量程上限"=w232, "测量值"=w228) -> ("数据标识"=w225:string)  [unwired: 7 in]
            n161 = Bundle By Name(cluster=w230, "数据标识mg/L"=w226, "数据标识%"=w225) -> (w227:T3)
            n162 = global write "多参数全局变量.vi" "DO2显示"(w227) -> ()
          }
          frame "Turb" {
            n163 = global read "断电保存变量.vi" "探头选择"() -> (w262:T7)
            n164 = Unbundle By Name(w262) -> ("浊度探头选择"=w261:T6)
            n165 = global read "多参数全局变量.vi" "MB session in"() -> (w260:refnum<class "MB_Master.lvclass">)
            n166 = case shown="\"STD\"" w261 {
              tunnel: w260 -> [w269 w277 w286 w290]
              tunnel: [w267 w275 w281 w291] -> w254
              tunnel: [w266 w274 w280 w289] -> w259
              frame "禹山", Default {
                n167 = call "禹山浊度_获取温度和测量值.vi"("MB session in"=w269) -> ("error out"=w266:errorcluster, "输出值"=w265:cluster{"温度测量值":sgl, "浊度":sgl})  [unwired: 8 in, 1 out]
                n168 = Unbundle By Name(w265) -> ("温度测量值"=w264:sgl, "浊度"=w263:sgl)
                n169 = global read "多参数全局变量.vi" "浊度显示"() -> (w268:T2)
                n170 = Bundle By Name(cluster=w268, "温度测量值"=w264, "测量值"=w263) -> (w267:T2)
              }
              frame "STD" {
                n171 = call "STD浊度_获取温度和测量值.vi"("MB session in"=w277) -> ("error out"=w274:errorcluster, "STD浊度"=w273:cluster{"温度测量值":sgl, "浊度测量值":sgl, "信号值":sgl})  [unwired: 8 in, 1 out]
                n172 = Unbundle By Name(w273) -> ("温度测量值"=w272:sgl, "浊度测量值"=w271:sgl, "信号值"=w270:sgl)
                n173 = global read "多参数全局变量.vi" "浊度显示"() -> (w276:T2)
                n174 = Bundle By Name(cluster=w276, "温度测量值"=w272, "测量值"=w271, "信号值"=w270) -> (w275:T2)
              }
              frame "国弘" {
                n175 = call "浊度_所有参数读取.vi"("MB session in"=w286) -> ("error out"=w280:errorcluster, "输出值"=w285:T14)  [unwired: 8 in, 1 out]
                n176 = Unbundle By Name(w285) -> ("温度测量值"=w283:sgl, "浊度测量值"=w282:sgl, "温度偏移修正值"=w279:sgl, "浊度信号值"=w278:sgl)
                n177 = global read "多参数全局变量.vi" "浊度显示"() -> (w284:T2)
                n178 = Bundle By Name(cluster=w284, "温度测量值"=w283, "测量值"=w282, "温度偏移修正值"=w279, "信号值"=w278) -> (w281:T2)
              }
              frame "纳清" {
                n179 = call "纳清浊度_所有参数读取.vi"("MB session in"=w290) -> ("error out"=w289:errorcluster, "输出值"=w288:T15)  [unwired: 8 in, 1 out]
                n180 = Unbundle By Name(w288) -> ("温度数据"=w293:sgl, "浊度数值 NTU"=w292:sgl, "原始光强数值"=w287:u16)
                n181 = global read "多参数全局变量.vi" "浊度显示"() -> (w294:T2)
                n182 = Bundle By Name(cluster=w294, "温度测量值"=w293, "测量值"=w292, "信号值"=w287) -> (w291:T2)
              }
            }
            n183 = global read "断电保存变量.vi" "量程参数"() -> (w258:T4)
            n184 = Unbundle By Name(w258) -> ("浊度 (NTU).量程上限"=w257:dbl, "浊度 (NTU).量程下限"=w256:dbl)
            n185 = Unbundle By Name(w254) -> ("测量值"=w253:sgl)
            n186 = Unbundle By Name(w259) -> ("status"=w255:bool)
            n187 = global write "多参数全局变量.vi" "浊度通讯状态"(w255) -> ()
            n188 = call "数据标识判定.vi"("通讯故障"=w255, "量程下限"=w256, "量程上限"=w257, "测量值"=w253) -> ("数据标识"=w251:string)  [unwired: 7 in]
            n189 = Bundle By Name(cluster=w254, "数据标识"=w251) -> (w252:T2)
            n190 = global write "多参数全局变量.vi" "浊度显示"(w252) -> ()
          }
          frame "悬浮物" {
            n191 = global read "断电保存变量.vi" "探头选择"() -> (w306:T7)
            n192 = Unbundle By Name(w306) -> ("悬浮物探头选择"=w305:T6)
            n193 = global read "多参数全局变量.vi" "MB session in"() -> (w304:refnum<class "MB_Master.lvclass">)
            n194 = case shown="\"STD\"" w305 {
              tunnel: w304 -> [_ w314]
              tunnel: [_ w312] -> w298
              tunnel: [_ w311] -> w303
              frame Default {
              }
              frame "STD" {
                n195 = call "STD悬浮物_获取温度和测量值.vi"("MB session in"=w314) -> ("error out"=w311:errorcluster, "STD浑浊度"=w310:cluster{"温度测量值":sgl, "悬浮物测量值":sgl, "信号值":sgl})  [unwired: 8 in, 1 out]
                n196 = Unbundle By Name(w310) -> ("温度测量值"=w309:sgl, "悬浮物测量值"=w308:sgl, "信号值"=w307:sgl)
                n197 = global read "多参数全局变量.vi" "悬浮物显示"() -> (w313:T2)
                n198 = Bundle By Name(cluster=w313, "温度测量值"=w309, "测量值"=w308, "信号值"=w307) -> (w312:T2)
              }
            }
            n199 = global read "断电保存变量.vi" "量程参数"() -> (w302:T4)
            n200 = Unbundle By Name(w302) -> ("悬浮物.量程上限"=w301:dbl, "悬浮物.量程下限"=w300:dbl)
            n201 = Unbundle By Name(w298) -> ("测量值"=w297:sgl)
            n202 = Unbundle By Name(w303) -> ("status"=w299:bool)
            n203 = global write "多参数全局变量.vi" "悬浮物通讯状态"(w299) -> ()
            n204 = call "数据标识判定.vi"("通讯故障"=w299, "量程下限"=w300, "量程上限"=w301, "测量值"=w297) -> ("数据标识"=w295:string)  [unwired: 7 in]
            n205 = Bundle By Name(cluster=w298, "数据标识"=w295) -> (w296:T2)
            n206 = global write "多参数全局变量.vi" "悬浮物显示"(w296) -> ()
          }
          frame "ORP" {
            n207 = global read "断电保存变量.vi" "探头选择"() -> (w326:T7)
            n208 = Unbundle By Name(w326) -> ("orp探头选择"=w325:T6)
            n209 = global read "多参数全局变量.vi" "MB session in"() -> (w324:refnum<class "MB_Master.lvclass">)
            n210 = case shown="\"禹山\", Default" w325 {
              tunnel: [_ w329 _] -> w323
              tunnel: w324 -> [_ w334 _]
              tunnel: [_ w327 _] -> w318
              frame "禹山", Default {
              }
              frame "国弘" {
                n211 = call "ORP_所有参数读取.vi"("MB session in"=w334) -> ("error out"=w329:errorcluster, "输出值"=w331:T16)  [unwired: 8 in, 1 out]
                n212 = Unbundle By Name(w331) -> ("温度测量值"=w332:sgl, "测量值"=w333:sgl, "信号值"=w328:sgl)
                n213 = global read "多参数全局变量.vi" "ORP显示"() -> (w330:T2)
                n214 = Bundle By Name(cluster=w330, "温度测量值"=w332, "测量值"=w333, "信号值"=w328) -> (w327:T2)
              }
              frame "纳清" {
              }
            }
            n215 = global read "断电保存变量.vi" "量程参数"() -> (w322:T4)
            n216 = Unbundle By Name(w322) -> ("ORP (mV).量程上限"=w321:dbl, "ORP (mV).量程下限"=w320:dbl)
            n217 = Unbundle By Name(w318) -> ("测量值"=w317:sgl)
            n218 = Unbundle By Name(w323) -> ("status"=w319:bool)
            n219 = global write "多参数全局变量.vi" "orp通讯状态"(w319) -> ()
            n220 = call "数据标识判定.vi"("通讯故障"=w319, "量程下限"=w320, "量程上限"=w321, "测量值"=w317) -> ("数据标识"=w315:string)  [unwired: 7 in]
            n221 = Bundle By Name(cluster=w318, "数据标识"=w315) -> (w316:T2)
            n222 = global write "多参数全局变量.vi" "ORP显示"(w316) -> ()
          }
          frame "叶绿素a" {
            n223 = global read "断电保存变量.vi" "探头选择"() -> (w346:T7)
            n224 = Unbundle By Name(w346) -> ("叶绿素a探头选择"=w345:T6)
            n225 = global read "多参数全局变量.vi" "MB session in"() -> (w344:refnum<class "MB_Master.lvclass">)
            n226 = case shown="\"STD\"" w345 {
              tunnel: [w353 w361 _ w367] -> w343
              tunnel: w344 -> [w352 w360 _ w369]
              tunnel: [w350 w358 _ w366] -> w339
              frame "禹山", Default {
                n227 = call "叶绿素a_获取温度和叶绿素值.vi"("MB session in"=w352) -> ("error out"=w353:errorcluster, "输出值"=w349:cluster{"温度测量值":sgl, "叶绿素测量值":sgl, "错误标志":u16})  [unwired: 8 in, 1 out]
                n228 = Unbundle By Name(w349) -> ("温度测量值"=w347:sgl, "叶绿素测量值"=w348:sgl)
                n229 = global read "多参数全局变量.vi" "叶绿素a显示"() -> (w351:T2)
                n230 = Bundle By Name(cluster=w351, "温度测量值"=w347, "测量值"=w348) -> (w350:T2)
              }
              frame "STD" {
                n231 = call "STDchla_获取温度和叶绿素值.vi"("MB session in"=w360) -> ("error out"=w361:errorcluster, "STD叶绿素a"=w357:cluster{"温度测量值":sgl, "叶绿素测量值":sgl, "信号值":sgl})  [unwired: 8 in, 1 out]
                n232 = Unbundle By Name(w357) -> ("温度测量值"=w355:sgl, "叶绿素测量值"=w356:sgl, "信号值"=w354:sgl)
                n233 = global read "多参数全局变量.vi" "叶绿素a显示"() -> (w359:T2)
                n234 = Bundle By Name(cluster=w359, "温度测量值"=w355, "测量值"=w356, "信号值"=w354) -> (w358:T2)
              }
              frame "国弘" {
              }
              frame "纳清" {
                n235 = call "纳清叶绿素a_所有参数读取.vi"("MB session in"=w369) -> ("error out"=w367:errorcluster, "输出值"=w365:T17)  [unwired: 8 in, 1 out]
                n236 = Unbundle By Name(w365) -> ("温度数据"=w363:sgl, "叶绿素a"=w364:sgl, "原始光强数值"=w362:u16)
                n237 = global read "多参数全局变量.vi" "叶绿素a显示"() -> (w368:T2)
                n238 = Bundle By Name(cluster=w368, "温度测量值"=w363, "测量值"=w364, "信号值"=w362) -> (w366:T2)
              }
            }
            n239 = global read "断电保存变量.vi" "量程参数"() -> (w342:T4)
            n240 = Unbundle By Name(w342) -> ("叶绿素a (μg/L).量程上限"=w341:dbl, "叶绿素a (μg/L).量程下限"=w340:dbl)
            n241 = Unbundle By Name(w339) -> ("测量值"=w338:sgl)
            n242 = Unbundle By Name(w343) -> ("status"=w337:bool)
            n243 = global write "多参数全局变量.vi" "叶绿素a通讯状态"(w337) -> ()
            n244 = call "数据标识判定.vi"("通讯故障"=w337, "量程下限"=w340, "量程上限"=w341, "测量值"=w338) -> ("数据标识"=w335:string)  [unwired: 7 in]
            n245 = Bundle By Name(cluster=w339, "数据标识"=w335) -> (w336:T2)
            n246 = global write "多参数全局变量.vi" "叶绿素a显示"(w336) -> ()
          }
          frame "藻密度" {
            n247 = global read "断电保存变量.vi" "探头选择"() -> (w381:T7)
            n248 = Unbundle By Name(w381) -> ("蓝绿藻探头选择"=w380:T6)
            n249 = global read "多参数全局变量.vi" "MB session in"() -> (w379:refnum<class "MB_Master.lvclass">)
            n250 = case shown="\"STD\"" w380 {
              tunnel: [_ w383 _ w395] -> w378
              tunnel: w379 -> [_ w384 _ w397]
              tunnel: [_ w382 _ w394] -> w374
              frame "禹山", Default {
              }
              frame "STD" {
                n251 = call "STDBGA_获取温度和叶绿素值.vi"("MB session in"=w384) -> ("error out"=w383:errorcluster, "STD藻密度"=w388:cluster{"温度测量值":sgl, "测试值":dbl, "信号值":sgl})  [unwired: 8 in, 1 out]
                n252 = Unbundle By Name(w388) -> ("温度测量值"=w386:sgl, "测试值"=w387:dbl, "信号值"=w385:sgl)
                n253 = global read "多参数全局变量.vi" "藻密度显示"() -> (w389:T2)
                n254 = Bundle By Name(cluster=w389, "温度测量值"=w386, "测量值"=w387, "信号值"=w385) -> (w382:T2)
              }
              frame "国弘" {
              }
              frame "纳清" {
                n255 = call "纳清蓝绿藻_所有参数读取.vi"("MB session in"=w397) -> ("error out"=w395:errorcluster, "输出值"=w393:T18)  [unwired: 8 in, 1 out]
                n256 = Unbundle By Name(w393) -> ("温度数据"=w392:sgl, "蓝绿藻"=w391:sgl, "原始光强数值"=w390:u16)
                n257 = global read "多参数全局变量.vi" "藻密度显示"() -> (w396:T2)
                n258 = Bundle By Name(cluster=w396, "温度测量值"=w392, "测量值"=w391, "信号值"=w390) -> (w394:T2)
              }
            }
            n259 = global read "断电保存变量.vi" "量程参数"() -> (w377:T4)
            n260 = Unbundle By Name(w377) -> ("藻密度 (cells/mL).量程上限"=w376:dbl, "藻密度 (cells/mL).量程下限"=w375:dbl)
            n261 = Unbundle By Name(w374) -> ("测量值"=w373:sgl)
            n262 = Unbundle By Name(w378) -> ("status"=w372:bool)
            n263 = global write "多参数全局变量.vi" "藻密度通讯状态"(w372) -> ()
            n264 = call "数据标识判定.vi"("通讯故障"=w372, "量程下限"=w375, "量程上限"=w376, "测量值"=w373) -> ("数据标识"=w370:string)  [unwired: 7 in]
            n265 = Bundle By Name(cluster=w374, "数据标识"=w370) -> (w371:T2)
            n266 = global write "多参数全局变量.vi" "藻密度显示"(w371) -> ()
          }
          frame "COD" {
            n267 = global read "断电保存变量.vi" "探头选择"() -> (w409:T7)
            n268 = Unbundle By Name(w409) -> ("COD探头选择"=w408:T6)
            n269 = global read "多参数全局变量.vi" "MB session in"() -> (w407:refnum<class "MB_Master.lvclass">)
            n270 = case shown="\"禹山\", Default" w408 {
              tunnel: [_ w415 _] -> w406
              tunnel: w407 -> [_ w417 _]
              tunnel: [_ w414 _] -> w405
              frame "禹山", Default {
              }
              frame "国弘" {
                n271 = call "COD_所有参数读取.vi"("MB session in"=w417) -> ("error out"=w415:errorcluster, "输出值"=w413:T19)  [unwired: 8 in, 1 out]
                n272 = Unbundle By Name(w413) -> ("温度测量值"=w412:sgl, "COD测量值"=w411:sgl, "COD信号值"=w410:sgl)
                n273 = global read "多参数全局变量.vi" "COD显示"() -> (w416:T2)
                n274 = Bundle By Name(cluster=w416, "温度测量值"=w412, "测量值"=w411, "信号值"=w410) -> (w414:T2)
              }
              frame "纳清" {
              }
            }
            n275 = global read "断电保存变量.vi" "量程参数"() -> (w400:T4)
            n276 = Unbundle By Name(w405) -> ("测量值"=w404:sgl)
            n277 = Unbundle By Name(w400) -> ("COD.量程上限"=w399:dbl, "COD.量程下限"=w398:dbl)
            n278 = Unbundle By Name(w406) -> ("status"=w403:bool)
            n279 = global write "多参数全局变量.vi" "cod通讯状态"(w403) -> ()
            n280 = call "数据标识判定.vi"("通讯故障"=w403, "量程下限"=w398, "量程上限"=w399, "测量值"=w404) -> ("数据标识"=w401:string)  [unwired: 7 in]
            n281 = Bundle By Name(cluster=w405, "数据标识"=w401) -> (w402:T2)
            n282 = global write "多参数全局变量.vi" "COD显示"(w402) -> ()
          }
          frame "氯化物" {
            n283 = global read "多参数全局变量.vi" "MB session in"() -> (w432:refnum<class "MB_Master.lvclass">)
            n284 = call "氯化物_所有参数读取.vi"("MB session in"=w432) -> ("error out"=w431:errorcluster, "输出值"=w424:T20)  [unwired: 8 in, 1 out]
            n285 = Unbundle By Name(w424) -> ("温度测量值"=w423:sgl, "测量值"=w422:sgl, "信号值"=w421:sgl)
            n286 = global read "多参数全局变量.vi" "氯化物显示"() -> (w425:T2)
            n287 = Unbundle By Name(w431) -> ("status"=w428:bool)
            n288 = global write "多参数全局变量.vi" "氯化物通讯状态"(w428) -> ()
            n289 = Bundle By Name(cluster=w425, "温度测量值"=w423, "测量值"=w422, "信号值"=w421) -> (w430:T2)
            n290 = global read "断电保存变量.vi" "量程参数"() -> (w420:T4)
            n291 = Unbundle By Name(w420) -> ("氯化物（mg/L）.量程上限"=w419:dbl, "氯化物（mg/L）.量程下限"=w418:dbl)
            n292 = Unbundle By Name(w430) -> ("测量值"=w429:sgl)
            n293 = call "数据标识判定.vi"("通讯故障"=w428, "量程下限"=w418, "量程上限"=w419, "测量值"=w429) -> ("数据标识"=w426:string)  [unwired: 7 in]
            n294 = Bundle By Name(cluster=w430, "数据标识"=w426) -> (w427:T2)
            n295 = global write "多参数全局变量.vi" "氯化物显示"(w427) -> ()
          }
          frame "水中油" {
            n296 = global read "多参数全局变量.vi" "MB session in"() -> (w435:refnum<class "MB_Master.lvclass">)
            n297 = call "水中油_所有参数读取.vi"("MB session in"=w435) -> ("error out"=w433:errorcluster, "输出值"=w434:T21)  [unwired: 8 in, 1 out]
            n298 = Unbundle By Name(w434) -> ("温度测量值"=w441:sgl, "测量值"=w440:sgl, "信号值"=w439:sgl)
            n299 = global read "多参数全局变量.vi" "水中油显示"() -> (w442:T2)
            n300 = Unbundle By Name(w433) -> ("status"=w445:bool)
            n301 = global write "多参数全局变量.vi" "水中油通讯状态"(w445) -> ()
            n302 = Bundle By Name(cluster=w442, "温度测量值"=w441, "测量值"=w440, "信号值"=w439) -> (w447:T2)
            n303 = global read "断电保存变量.vi" "量程参数"() -> (w438:T4)
            n304 = Unbundle By Name(w438) -> ("水中油.量程上限"=w437:dbl, "水中油.量程下限"=w436:dbl)
            n305 = Unbundle By Name(w447) -> ("测量值"=w446:sgl)
            n306 = call "数据标识判定.vi"("通讯故障"=w445, "量程下限"=w436, "量程上限"=w437, "测量值"=w446) -> ("数据标识"=w443:string)  [unwired: 7 in]
            n307 = Bundle By Name(cluster=w447, "数据标识"=w443) -> (w444:T2)
            n308 = global write "多参数全局变量.vi" "水中油显示"(w444) -> ()
          }
          frame "余氯" {
            n309 = global read "多参数全局变量.vi" "MB session in"() -> (w450:refnum<class "MB_Master.lvclass">)
            n310 = call "纳清余氯_所有参数读取.vi"("MB session in"=w450) -> ("error out"=w449:errorcluster, "输出值"=w448:T22)  [unwired: 8 in, 1 out]
            n311 = Unbundle By Name(w448) -> ("温度值"=w456:sgl, "余氯值"=w455:sgl, "氯电压_mv"=w454:dbl)
            n312 = Unbundle By Name(w449) -> ("status"=w460:bool)
            n313 = global read "多参数全局变量.vi" "余氯显示"() -> (w457:T2)
            n314 = global write "多参数全局变量.vi" "余氯通讯状态"(w460) -> ()
            n315 = Bundle By Name(cluster=w457, "温度测量值"=w456, "测量值"=w455, "信号值"=w454) -> (w462:T2)
            n316 = global read "断电保存变量.vi" "量程参数"() -> (w453:T4)
            n317 = Unbundle By Name(w462) -> ("测量值"=w461:sgl)
            n318 = Unbundle By Name(w453) -> ("余氯.量程上限"=w452:dbl, "余氯.量程下限"=w451:dbl)
            n319 = call "数据标识判定.vi"("通讯故障"=w460, "量程下限"=w451, "量程上限"=w452, "测量值"=w461) -> ("数据标识"=w458:string)  [unwired: 7 in]
            n320 = Bundle By Name(cluster=w462, "数据标识"=w458) -> (w459:T2)
            n321 = global write "多参数全局变量.vi" "余氯显示"(w459) -> ()
          }
          frame "氨氮" {
            n322 = global read "多参数全局变量.vi" "MB session in"() -> (w465:refnum<class "MB_Master.lvclass">)
            n323 = call "纳清氨氮_所有参数读取.vi"("MB session in"=w465) -> ("error out"=w463:errorcluster, "输出值"=w464:T23)  [unwired: 8 in, 1 out]
            n324 = Unbundle By Name(w464) -> ("温度数据"=w471:sgl, "参数2数据"=w470:sgl, "参数2原始信号"=w469:sgl)
            n325 = Unbundle By Name(w463) -> ("status"=w475:bool)
            n326 = global read "多参数全局变量.vi" "氨氮显示"() -> (w472:T2)
            n327 = global write "多参数全局变量.vi" "氨氮通讯状态"(w475) -> ()
            n328 = Bundle By Name(cluster=w472, "温度测量值"=w471, "测量值"=w470, "信号值"=w469) -> (w477:T2)
            n329 = global read "断电保存变量.vi" "量程参数"() -> (w468:T4)
            n330 = Unbundle By Name(w477) -> ("测量值"=w476:sgl)
            n331 = Unbundle By Name(w468) -> ("氨氮.量程上限"=w467:dbl, "氨氮.量程下限"=w466:dbl)
            n332 = call "数据标识判定.vi"("通讯故障"=w475, "量程下限"=w466, "量程上限"=w467, "测量值"=w476) -> ("数据标识"=w473:string)  [unwired: 7 in]
            n333 = Bundle By Name(cluster=w477, "数据标识"=w473) -> (w474:T2)
            n334 = global write "多参数全局变量.vi" "氨氮显示"(w474) -> ()
          }
        }
      }
      frame #2 {
        n335 = Format Date/Time String() -> (date/time string=→"日期/时间字符串 2":string)  [unwired: 3 in]
        n336 = Wait (ms)(milliseconds to wait=u32 500 ("等待时间（毫秒）")) -> ()  [unwired: 1 out]
      }
    }
  }
  n337 = while {
    tunnel: w1 -> [w689]
    stop <- FALSE stop-if-true
    w589 = T1[] [enum."pH", enum."DO", enum."Cond", enum."Turb", enum."ORP", enum."叶绿素a", enum."藻密度", enum."COD", enum."DO2", enum."氯化物", enum."氨氮", enum."水中油", enum."悬浮物", enum."余氯"] items=["pH", "DO", "DO2", "Cond", "Turb", "ORP", "叶绿素a", "藻密度", "COD", "氯化物", "氨氮", "水中油", "悬浮物", "余氯"]
    n338 = global read "多参数全局变量.vi" "远程校准运行状态"() -> (w686:T24)
    n339 = global read "多参数全局变量.vi" "远程校准运行状态"() -> (w660:T24)
    n340 = global read "多参数全局变量.vi" "远程校准运行状态"() -> (w663:T24)
    n341 = global read "多参数全局变量.vi" "远程校准运行状态"() -> (w647:T24)
    n342 = global read "多参数全局变量.vi" "远程校准运行状态"() -> (w634:T24)
    n343 = global read "多参数全局变量.vi" "远程校准运行状态"() -> (w577:T24)
    n344 = global read "多参数全局变量.vi" "远程校准运行状态"() -> (w559:T24)
    n345 = global read "多参数全局变量.vi" "远程校准运行状态"() -> (w523:T24)
    n346 = global read "多参数全局变量.vi" "远程校准运行状态"() -> (w495:T24)
    n347 = global read "多参数全局变量.vi" "远程校准运行状态"() -> (w493:T24)
    n348 = global read "多参数全局变量.vi" "校准运行状态"() -> (w675:T25)
    n349 = global read "多参数全局变量.vi" "校准运行状态"() -> (w649:T25)
    n350 = global read "多参数全局变量.vi" "校准运行状态"() -> (w674:T25)
    n351 = global read "多参数全局变量.vi" "校准运行状态"() -> (w636:T25)
    n352 = global read "多参数全局变量.vi" "校准运行状态"() -> (w623:T25)
    n353 = global read "多参数全局变量.vi" "校准运行状态"() -> (w584:T25)
    n354 = global read "多参数全局变量.vi" "校准运行状态"() -> (w570:T25)
    n355 = global read "多参数全局变量.vi" "校准运行状态"() -> (w534:T25)
    n356 = global read "多参数全局变量.vi" "校准运行状态"() -> (w506:T25)
    n357 = global read "多参数全局变量.vi" "校准运行状态"() -> (w482:T25)
    n358 = global read "多参数全局变量.vi" "远程校准运行状态"() -> (w611:T24)
    n359 = global read "多参数全局变量.vi" "远程校准运行状态"() -> (w608:T24)
    n360 = global read "多参数全局变量.vi" "远程校准运行状态"() -> (w549:T24)
    n361 = global read "多参数全局变量.vi" "远程校准运行状态"() -> (w521:T24)
    n362 = global read "多参数全局变量.vi" "校准运行状态"() -> (w622:T25)
    n363 = global read "多参数全局变量.vi" "校准运行状态"() -> (w597:T25)
    n364 = global read "多参数全局变量.vi" "校准运行状态"() -> (w538:T25)
    n365 = global read "多参数全局变量.vi" "校准运行状态"() -> (w510:T25)
    n366 = Unbundle By Name(w506) -> ("悬浮物"=w504:bool)
    n367 = Unbundle By Name(w495) -> ("悬浮物"=w497:bool)
    n368 = Unbundle By Name(w674) -> ("Cond"=w672:bool)
    n369 = Unbundle By Name(w663) -> ("Cond"=w664:bool)
    n370 = Unbundle By Name(w636) -> ("Turb"=w638:bool)
    n371 = Unbundle By Name(w647) -> ("Turb"=w646:bool)
    n372 = Unbundle By Name(w584) -> ("COD"=w583:bool)
    n373 = Unbundle By Name(w623) -> ("ORP"=w625:bool)
    n374 = Unbundle By Name(w634) -> ("ORP"=w633:bool)
    n375 = Unbundle By Name(w570) -> ("DO2"=w568:bool)
    n376 = Unbundle By Name(w559) -> ("DO2"=w560:bool)
    n377 = Unbundle By Name(w534) -> ("氨氮"=w532:bool)
    n378 = Unbundle By Name(w523) -> ("氨氮"=w525:bool)
    n379 = Unbundle By Name(w482) -> ("余氯"=w484:bool)
    n380 = Unbundle By Name(w493) -> ("余氯"=w491:bool)
    n381 = Unbundle By Name(w649) -> ("DO"=w651:bool)
    n382 = Unbundle By Name(w660) -> ("DO"=w659:bool)
    n383 = Unbundle By Name(w577) -> ("cod"=w578:bool)
    n384 = Unbundle By Name(w675) -> ("ph"=w677:bool)
    n385 = Unbundle By Name(w686) -> ("ph"=w685:bool)
    n386 = Cluster To Array(cluster=w675) -> (array=w680:bool[])
    n387 = Cluster To Array(cluster=w686) -> (array=w682:bool[])
    n388 = Cluster To Array(cluster=w649) -> (array=w654:bool[])
    n389 = Cluster To Array(cluster=w660) -> (array=w656:bool[])
    n390 = Cluster To Array(cluster=w674) -> (array=w669:bool[])
    n391 = Cluster To Array(cluster=w663) -> (array=w667:bool[])
    n392 = Cluster To Array(cluster=w636) -> (array=w641:bool[])
    n393 = Cluster To Array(cluster=w647) -> (array=w643:bool[])
    n394 = Cluster To Array(cluster=w623) -> (array=w628:bool[])
    n395 = Cluster To Array(cluster=w634) -> (array=w630:bool[])
    n396 = Cluster To Array(cluster=w584) -> (array=w580:bool[])
    n397 = Cluster To Array(cluster=w577) -> (array=w576:bool[])
    n398 = Cluster To Array(cluster=w570) -> (array=w565:bool[])
    n399 = Cluster To Array(cluster=w559) -> (array=w563:bool[])
    n400 = Cluster To Array(cluster=w534) -> (array=w533:bool[])
    n401 = Cluster To Array(cluster=w523) -> (array=w524:bool[])
    n402 = Cluster To Array(cluster=w506) -> (array=w505:bool[])
    n403 = Cluster To Array(cluster=w495) -> (array=w496:bool[])
    n404 = Cluster To Array(cluster=w482) -> (array=w483:bool[])
    n405 = Cluster To Array(cluster=w493) -> (array=w492:bool[])
    n406 = Unbundle By Name(w622) -> ("叶绿素a"=w620:bool)
    n407 = Unbundle By Name(w611) -> ("叶绿素a"=w612:bool)
    n408 = Unbundle By Name(w597) -> ("藻密度"=w599:bool)
    n409 = Unbundle By Name(w608) -> ("藻密度"=w607:bool)
    n410 = Unbundle By Name(w538) -> ("氯化物"=w540:bool)
    n411 = Unbundle By Name(w549) -> ("氯化物"=w547:bool)
    n412 = Unbundle By Name(w510) -> ("水中油"=w512:bool)
    n413 = Unbundle By Name(w521) -> ("水中油"=w519:bool)
    n414 = Boolean Array To Number(Boolean array=w680) -> (number=w679:u32)
    n415 = Boolean Array To Number(Boolean array=w682) -> (number=w683:u32)
    n416 = Boolean Array To Number(Boolean array=w654) -> (number=w653:u32)
    n417 = Boolean Array To Number(Boolean array=w656) -> (number=w657:u32)
    n418 = Boolean Array To Number(Boolean array=w669) -> (number=w670:u32)
    n419 = Boolean Array To Number(Boolean array=w667) -> (number=w666:u32)
    n420 = Boolean Array To Number(Boolean array=w641) -> (number=w640:u32)
    n421 = Boolean Array To Number(Boolean array=w643) -> (number=w644:u32)
    n422 = Boolean Array To Number(Boolean array=w628) -> (number=w627:u32)
    n423 = Boolean Array To Number(Boolean array=w630) -> (number=w631:u32)
    n424 = Boolean Array To Number(Boolean array=w580) -> (number=w581:u32)
    n425 = Boolean Array To Number(Boolean array=w576) -> (number=w575:u32)
    n426 = Boolean Array To Number(Boolean array=w565) -> (number=w566:u32)
    n427 = Boolean Array To Number(Boolean array=w563) -> (number=w562:u32)
    n428 = Boolean Array To Number(Boolean array=w533) -> (number=w531:u32)
    n429 = Boolean Array To Number(Boolean array=w524) -> (number=w526:u32)
    n430 = Boolean Array To Number(Boolean array=w505) -> (number=w503:u32)
    n431 = Boolean Array To Number(Boolean array=w496) -> (number=w498:u32)
    n432 = Boolean Array To Number(Boolean array=w483) -> (number=w485:u32)
    n433 = Boolean Array To Number(Boolean array=w492) -> (number=w490:u32)
    n434 = Cluster To Array(cluster=w622) -> (array=w617:bool[])
    n435 = Cluster To Array(cluster=w611) -> (array=w615:bool[])
    n436 = Cluster To Array(cluster=w597) -> (array=w602:bool[])
    n437 = Cluster To Array(cluster=w608) -> (array=w604:bool[])
    n438 = Cluster To Array(cluster=w538) -> (array=w539:bool[])
    n439 = Cluster To Array(cluster=w549) -> (array=w548:bool[])
    n440 = Cluster To Array(cluster=w510) -> (array=w511:bool[])
    n441 = Cluster To Array(cluster=w521) -> (array=w520:bool[])
    n442 = Equal To 0?(x=w679) -> (x = 0?=w678:bool)
    n443 = Equal To 0?(x=w683) -> (x = 0?=w684:bool)
    n444 = Equal To 0?(x=w653) -> (x = 0?=w652:bool)
    n445 = Equal To 0?(x=w657) -> (x = 0?=w658:bool)
    n446 = Equal To 0?(x=w670) -> (x = 0?=w671:bool)
    n447 = Equal To 0?(x=w666) -> (x = 0?=w665:bool)
    n448 = Equal To 0?(x=w640) -> (x = 0?=w639:bool)
    n449 = Equal To 0?(x=w644) -> (x = 0?=w645:bool)
    n450 = Equal To 0?(x=w627) -> (x = 0?=w626:bool)
    n451 = Equal To 0?(x=w631) -> (x = 0?=w632:bool)
    n452 = Equal To 0?(x=w581) -> (x = 0?=w582:bool)
    n453 = Equal To 0?(x=w575) -> (x = 0?=w579:bool)
    n454 = Equal To 0?(x=w566) -> (x = 0?=w567:bool)
    n455 = Equal To 0?(x=w562) -> (x = 0?=w561:bool)
    n456 = Equal To 0?(x=w531) -> (x = 0?=w530:bool)
    n457 = Equal To 0?(x=w526) -> (x = 0?=w527:bool)
    n458 = Equal To 0?(x=w503) -> (x = 0?=w502:bool)
    n459 = Equal To 0?(x=w498) -> (x = 0?=w499:bool)
    n460 = Equal To 0?(x=w485) -> (x = 0?=w486:bool)
    n461 = Equal To 0?(x=w490) -> (x = 0?=w489:bool)
    n462 = Boolean Array To Number(Boolean array=w617) -> (number=w618:u32)
    n463 = Boolean Array To Number(Boolean array=w615) -> (number=w614:u32)
    n464 = Boolean Array To Number(Boolean array=w602) -> (number=w601:u32)
    n465 = Boolean Array To Number(Boolean array=w604) -> (number=w605:u32)
    n466 = Boolean Array To Number(Boolean array=w539) -> (number=w541:u32)
    n467 = Boolean Array To Number(Boolean array=w548) -> (number=w546:u32)
    n468 = Boolean Array To Number(Boolean array=w511) -> (number=w513:u32)
    n469 = Boolean Array To Number(Boolean array=w520) -> (number=w518:u32)
    n470 = Or(x=w677, y=w678) -> (x .or. y?=w676:bool)
    n471 = Or(x=w685, y=w684) -> (x .or. y?=w687:bool)
    n472 = Or(x=w651, y=w652) -> (x .or. y?=w650:bool)
    n473 = Or(x=w659, y=w658) -> (x .or. y?=w661:bool)
    n474 = Or(x=w672, y=w671) -> (x .or. y?=w673:bool)
    n475 = Or(x=w664, y=w665) -> (x .or. y?=w662:bool)
    n476 = Or(x=w638, y=w639) -> (x .or. y?=w637:bool)
    n477 = Or(x=w646, y=w645) -> (x .or. y?=w648:bool)
    n478 = Or(x=w625, y=w626) -> (x .or. y?=w624:bool)
    n479 = Or(x=w633, y=w632) -> (x .or. y?=w635:bool)
    n480 = Or(x=w583, y=w582) -> (x .or. y?=w574:bool)
    n481 = Or(x=w578, y=w579) -> (x .or. y?=w573:bool)
    n482 = Or(x=w568, y=w567) -> (x .or. y?=w569:bool)
    n483 = Or(x=w560, y=w561) -> (x .or. y?=w558:bool)
    n484 = Or(x=w532, y=w530) -> (x .or. y?=w535:bool)
    n485 = Or(x=w525, y=w527) -> (x .or. y?=w529:bool)
    n486 = Or(x=w504, y=w502) -> (x .or. y?=w507:bool)
    n487 = Or(x=w497, y=w499) -> (x .or. y?=w501:bool)
    n488 = Or(x=w484, y=w486) -> (x .or. y?=w481:bool)
    n489 = Or(x=w491, y=w489) -> (x .or. y?=w487:bool)
    n490 = Equal To 0?(x=w618) -> (x = 0?=w619:bool)
    n491 = Equal To 0?(x=w614) -> (x = 0?=w613:bool)
    n492 = Equal To 0?(x=w601) -> (x = 0?=w600:bool)
    n493 = Equal To 0?(x=w605) -> (x = 0?=w606:bool)
    n494 = Equal To 0?(x=w541) -> (x = 0?=w542:bool)
    n495 = Equal To 0?(x=w546) -> (x = 0?=w545:bool)
    n496 = Equal To 0?(x=w513) -> (x = 0?=w514:bool)
    n497 = Equal To 0?(x=w518) -> (x = 0?=w517:bool)
    n498 = global read "断电保存变量.vi" "叶绿素a启用"() -> (w616:bool)
    n499 = global read "断电保存变量.vi" "藻密度"() -> (w603:bool)
    n500 = global read "断电保存变量.vi" "氯化物"() -> (w544:bool)
    n501 = global read "断电保存变量.vi" "水中油"() -> (w516:bool)
    n502 = global read "断电保存变量.vi" "Cond"() -> (w668:bool)
    n503 = global read "断电保存变量.vi" "DO 2"() -> (w564:bool)
    n504 = global read "断电保存变量.vi" "Turb"() -> (w642:bool)
    n505 = global read "断电保存变量.vi" "COD"() -> (w585:bool)
    n506 = Or(x=w620, y=w619) -> (x .or. y?=w621:bool)
    n507 = Or(x=w612, y=w613) -> (x .or. y?=w610:bool)
    n508 = Or(x=w599, y=w600) -> (x .or. y?=w598:bool)
    n509 = Or(x=w607, y=w606) -> (x .or. y?=w609:bool)
    n510 = Or(x=w540, y=w542) -> (x .or. y?=w537:bool)
    n511 = Or(x=w547, y=w545) -> (x .or. y?=w543:bool)
    n512 = global read "断电保存变量.vi" "氨氮"() -> (w528:bool)
    n513 = Or(x=w512, y=w514) -> (x .or. y?=w509:bool)
    n514 = Or(x=w519, y=w517) -> (x .or. y?=w515:bool)
    n515 = global read "断电保存变量.vi" "余氯"() -> (w488:bool)
    n516 = global read "断电保存变量.vi" "orp"() -> (w629:bool)
    n517 = global read "断电保存变量.vi" "DO"() -> (w655:bool)
    n518 = global read "断电保存变量.vi" "pH"() -> (w681:bool)
    n519 = global read "断电保存变量.vi" "SS"() -> (w500:bool)
    n520 = Compound Arithmetic op=AND ("复合运算")(w681, w676, w687) -> (w596:bool)
    n521 = Compound Arithmetic op=AND ("复合运算")(w655, w650, w661) -> (w571:bool)
    n522 = Compound Arithmetic op=AND ("复合运算")(w668, w673, w662) -> (w595:bool)
    n523 = Compound Arithmetic op=AND ("复合运算")(w642, w637, w648) -> (w594:bool)
    n524 = Compound Arithmetic op=AND ("复合运算")(w629, w624, w635) -> (w593:bool)
    n525 = Compound Arithmetic op=AND ("复合运算")(w616, w621, w610) -> (w592:bool)
    n526 = Compound Arithmetic op=AND ("复合运算")(w603, w598, w609) -> (w591:bool)
    n527 = Compound Arithmetic op=AND ("复合运算")(w585, w574, w573) -> (w572:bool)
    n528 = Compound Arithmetic op=AND ("复合运算")(w564, w569, w558) -> (w557:bool)
    n529 = Compound Arithmetic op=AND ("复合运算")(w544, w537, w543) -> (w536:bool)
    n530 = Compound Arithmetic op=AND ("复合运算")(w528, w535, w529) -> (w522:bool)
    n531 = Compound Arithmetic op=AND ("复合运算")(w516, w509, w515) -> (w508:bool)
    n532 = Compound Arithmetic op=AND ("复合运算")(w500, w507, w501) -> (w494:bool)
    n533 = Compound Arithmetic op=AND ("复合运算")(w488, w481, w487) -> (w480:bool)
    n534 = Build Array(w596, w571, w595, w594, w593, w592, w591, w572, w557, w536, w522, w508, w494, w480) -> (w590:bool[])
    n535 = for {
      tunnel: w590 -> [w695] mode=indexing
      tunnel: w589 -> [w696] mode=indexing
      tunnel: [w696] -> w588 mode=indexing if=w695
      tunnel: [w694] -> w556
      i -> [w694]
    }
    n536 = Less Or Equal?(x=w556, y=1) -> (x <= y?=w554:bool)
    n537 = Select(t=u32 2000 ("等待时间（毫秒）"), s=w554, f=u32 1000 ("等待时间（毫秒）")) -> (s? t:f=w551:u32)
    n538 = Wait (ms)(milliseconds to wait=w551) -> (millisecond timer value=w550:u32)
    n539 = Get Queue Status(queue=w689) -> (queue out=w587:refnum<queue>, # elements in queue=w586:i32)  [unwired: 2 in, 6 out]
    n540 = case shown="0" w586 {
      tunnel: w588 -> [_ w691]
      tunnel: w587 -> [_ w690]
      tunnel: w550 -> [_ _]
      frame Default {
      }
      frame 0 {
        n541 = for {
          tunnel: w690 -> [w693]
          tunnel: w691 -> [w692] mode=indexing
          n542 = Enqueue Element(queue=w693, element=w692) -> ()  [unwired: 2 in, 3 out]
        }
      }
    }
  }
